vi "Dashboard custom_bartender&global&gripper&camera4.vi"() -> ()   [LabVIEW 2017]
uses:
  C:/Users/IMR Lab/Documents/LabVIEW Data/UniversalRobotsSDK_LABView/LabVIEW/Examples/LabVIEW10/UnderAutomation.UniversalRobots.dll
  UnderAutomation.UniversalRobots.dll
  Global 1.vi
panel:
  in  "stop":bool
  out "3rd Order":bool
  out "2nd Order":bool
  out "1st Order":bool
  out "Rx":dbl
  out "Rz":dbl
  out "Ry":dbl
  out "Enabled":bool
  out "Port":i32
  in  "Move to particular posture":bool
  in  "Move to Zero position":bool
  out "Connected":bool
  in  "Robot IP(192.168.112.182)":string
  out "Connect error":errorcluster
  in  "Power on\nRelease brake":bool
  in  "Power off":bool
  in  "Connect":bool
  in  "Send script":bool
  in  "Script to execute":string
  out "Powered on":bool
  out "X":dbl
  out "Y":dbl
  out "Z":dbl
  out "License state":string
  # "e"
  # "movej( get_inverse_kin(p[0.3138, 0.0814, 0.1647, 0.4226, -2.3876, -2.3851]),  a=0.5, v=0.25, t=0, r=0)"
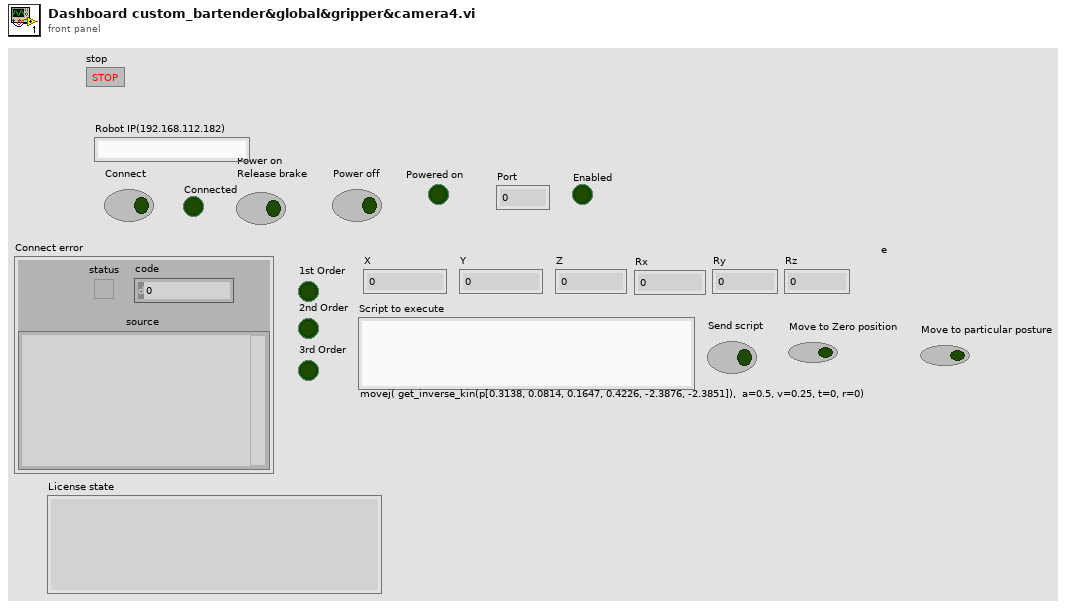
[diagram p1: front panel]
types:
  T1 = enum16{"Standard", "Buffered", "CRLF", "Immediate"}
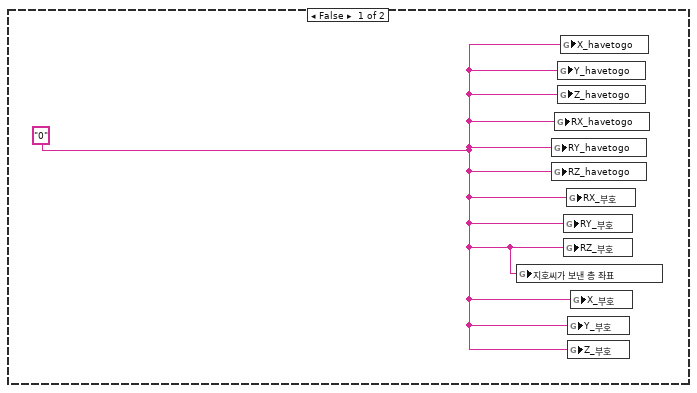
[diagram p2: hidden frame]
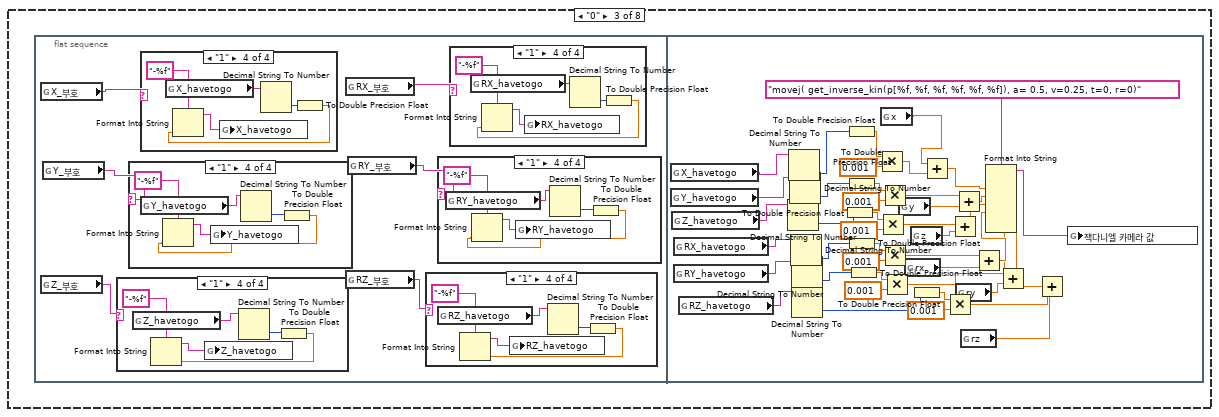
[diagram p5: hidden frame]
diagram:
  w6 = ""
  # "짐빔에서 우유이동 준비 자세"
  # "우유 들어올리는 자세"
  # "우유로 가는 자세"
  # "우유 보는 자세"
  # "술잔 따르는 자세3"
  # "미니콜라 따르는 자세"
  # "술잔 중간지점 가는 자세"
  # "짐빔에서 토닉이동 준비 자세"
  # "술잔 따르는 자세2"
  # "술잔 위로 가는 자세2"
  # "토닉워터 뺴는 자세"
  # "토닉워 들어올리는 자세"
  # "토닉워터 가는 자세"
  # "토닉워터 보는 자세"
  # "짐빔 들어올리는 자세"
  # "짐빔로 가는 자세"
  # "짐빔 보는 자세"
  # "콜라 뺴는 자세"
  # "콜라 들어올리는 자세"
  # "콜라로 가는 자세"
  # "콜라 보는 자세"
  # "술잔 따르는 자세"
  # "술잔 위로 가는 자세"
  # "잭다니엘 들어올리는 자세"
  # "잭다니엘 위치로 가는 자세"
  # "잭다니엘 보는 자세"
  # "1자로 서는 자세"
  # "Example : Display power on status"
  # "Create a UR\ncobot instance"
  # "Show license state"
  # "Register your confidential license key to exit\ntrial period and use this library forever"
  # "Power off when button is clicked"
  # "Power on and release brake when button is clicked"
  # "Get your UR Dashboard interface"
  n1 = global write "Global 1.vi" "술따르는자세2-2"("movej( get_inverse_kin(p[-0.114997, -0.200333, 0.241627, 0.772074, 1.70292, -1.57709]), a= 0.5, v=0.25, t=0, r=0)") -> ()
  n2 = global write "Global 1.vi" "TCP 스위치"(FALSE ("TCP 스위치")) -> ()
  n3 = global write "Global 1.vi" "미니콜라 따르는 자세"("movej([-0.0902,-1.8120,-1.9241,-3.5769,6.2827,8.4658], a=0.5, v=0.25, t=0, r=0)") -> ()
  n4 = global write "Global 1.vi" "짐빔에서 우유준비자세"("movej( get_inverse_kin(p[-0.226891, 0.162413, 0.418489, -0.313613, 2.00693, 1.9348]), a= 0.5, v=0.25, t=0, r=0)") -> ()
  n5 = global write "Global 1.vi" "잭다니엘 들어올리는 자세"("movej([0.8116,-2.0223,-1.2828,-3.0107,4.3284,5.9341], a=0.5, v=0.25, t=0, r=0)") -> ()
  n6 = global write "Global 1.vi" "짐빔 토닉 이동 준비자세"("movej([-0.5421,-0.8131,0.8439,-0.0538,2.5052,5.9032], a=0.5, v=0.25, t=0, r=0)") -> ()
  n7 = global write "Global 1.vi" "우유로 가는 자세"("movej( get_inverse_kin(p[-0.0922578, 0.258702, 0.0945584, -0.185663, 1.9856, 1.89851]), a= 0.5, v=0.25, t=0, r=0)") -> ()
  n8 = global write "Global 1.vi" "우유드는자세"("movej( get_inverse_kin(p[-0.0942522, 0.213042, 0.40064, -0.176149, 1.92162, 1.97243]), a= 0.5, v=0.25, t=0, r=0)") -> ()
  n9 = global write "Global 1.vi" "우유보는자세"("movej( get_inverse_kin(p[-0.103424, 0.183937, 0.100861, -0.211125, 2.02982, 1.84622]), a= 0.5, v=0.25, t=0, r=0)") -> ()
  n10 = global write "Global 1.vi" "토닉 빼는 자세"("movej([-0.5277,-1.5104,1.5889,-0.0548,2.5728,5.9025], a=0.5, v=0.25, t=0, r=0)") -> ()
  n11 = global write "Global 1.vi" "잭다닐 위치로 가는 자세"("movej([0.8116,-2.3119,-1.606,-2.3958,4.3284,5.9341], a=0.5, v=0.25, t=0, r=0)") -> ()
  n12 = global write "Global 1.vi" "토닉 드는 자세"("movej([-1.0311,-1.1460,1.5830,-0.4348,2.0708,5.9048], a=0.5, v=0.25, t=0, r=0)") -> ()
  n13 = global write "Global 1.vi" "토닉 보는 자세"("movej([-0.4690,-1.1292,2.1508,-1.0119,2.6124,5.9032], a=0.5, v=0.25, t=0, r=0)") -> ()
  n14 = global write "Global 1.vi" "술잔 위로 가는 자세 2"("movej([0.0485,-1.6015,2.5780,-1.0382,-0.0520,5.3649], a=0.5, v=0.25, t=0, r=0)") -> ()
  n15 = global write "Global 1.vi" "1자로 서는 자세"("movej([3.1412,-1.5708,0,-1.5708,3.1412,5.8904], a=0.5, v=0.25, t=0, r=0)") -> ()
  n16 = global write "Global 1.vi" "짐빔 들어올리는 자세"("movej([-0.5421,-0.8131,0.8439,-0.0538,2.5052,5.9032], a=0.5, v=0.25, t=0, r=0)") -> ()
  n17 = global write "Global 1.vi" "술잔 위로 가는 자세"("movej([-0.0903,-2.0548,-2.0169,-3.3289,6.2826,7.4091], a=0.5, v=0.25, t=0, r=0)") -> ()
  n18 = global write "Global 1.vi" "토닉 가는자세"("movej([-0.9924,-0.8742,1.7459,-0.8837,2.0958,5.9048], a=0.5, v=0.25, t=0, r=0)") -> ()
  n19 = global write "Global 1.vi" "잭다니엘 보는 자세"("movej([0,-2.2170,-1.4226,-2.2842,3.1412,6.2832], a=0.5, v=0.25, t=0, r=0)") -> ()
  n20 = global write "Global 1.vi" "짐빔 위치로 가는 자세"("movej([-0.5436,-0.4519,0.8428,-0.3534,2.6134,5.9032], a=0.5, v=0.25, t=0, r=0)") -> ()
  n21 = global write "Global 1.vi" "콜라 보는 자세"("movej([0,-1.8110,-2.1684,-2.3033,3.1543,5.9213], a=0.5, v=0.25, t=0, r=0)") -> ()
  n22 = global write "Global 1.vi" "콜라로 가는자세"("movej([1.2020,-2.166,-1.9385,-2.1863,4.3172,5.9210], a=0.5, v=0.25, t=0, r=0)") -> ()
  n23 = global write "Global 1.vi" "콜라 빼는 자세"("movej([0.8789,-1.5237,-2.1070,-2.6679, 3.9917,5.9085], a=0.5, v=0.25, t=0, r=0)") -> ()
  n24 = global write "Global 1.vi" "콜라 드는 자세"("movej([1.2020,-1.8452,-1.7403,-2.7082,4.3162,5.9158], a=0.5, v=0.25, t=0, r=0)") -> ()
  n25 = global write "Global 1.vi" "술 따르는 자세 2"("movej([0.0412,-1.9708,2.4700,-1.0157,-0.0618,4.8998], a=0.5, v=0.25, t=0, r=0)") -> ()
  n26 = global write "Global 1.vi" "잭다니엘 카메라 값"(w6) -> ()
  n27 = global write "Global 1.vi" "술 따르는 자세"("movej([-0.0902,-1.9024,-1.9241,-3.5769,6.2827,8.4692], a=0.5, v=0.25, t=0, r=0)") -> ()
  n28 = global write "Global 1.vi" "짐빔 보는 자세"("movej([-0.0364,-0.6154,0.9421,-0.3291,3.1047,5.9020], a=0.5, v=0.25, t=0, r=0)") -> ()
  n29 = global write "Global 1.vi" "콜라 카메라 값"(w6) -> ()
  n30 = global write "Global 1.vi" "토닉 카메라 값"(w6) -> ()
  n31 = global write "Global 1.vi" "짐빔 카메라 값"(w6) -> ()
  n32 = constructor class="UR"() -> (reference out=w32:refnum<k24>)  [unwired: 3 in, 2 out]
  n33 = global write "Global 1.vi" "술잔 중간지점"("movej([-0.2173,-1.9485,-1.6874,-3.9352,6.2671,7.2276], a=0.5, v=0.25, t=0, r=0)") -> ()
  n34 = while {
    tunnel: w32 -> [w38]
    stop <- FALSE stop-if-true
    # "Connect to the robot when button is pressed"
    # "Show if primary interface is connected"
    # "Get your UR primary interface"
    n35 = property class="UR"(reference=w38) -> ("PrimaryInterface"=w41:refnum<k24>)  [unwired: 1 in, 2 out]
    n36 = Wait (ms)(milliseconds to wait=u32 50) -> ()  [unwired: 1 out]
    n37 = property class="PrimaryInterfaceClientInternal"(reference=w41) -> ("Connected"=w40:bool)  [unwired: 1 in, 2 out]
    "Connected" <- w40
    n38 = case shown="True" "Connect" {
      tunnel: w38 -> [_ w708]
      frame False {
      }
      frame True {
        n39 = flat-sequence {
          tunnel: w708 -> [w710]
          frame #0 {
            n40 = invoke class="UR" method="Connect"(reference=w710, "ip"="Robot IP(192.168.112.182)") -> (error out=→"Connect error":errorcluster)  [unwired: 2 in, 3 out]
          }
        }
      }
    }
    n41 = case shown="True" w40 {
      tunnel: w41 -> [_ w54]
      frame False {
        (unwired) 0.0 ("Rx")
        (unwired) 0.0 ("Rz")
        (unwired) 0.0 ("Ry")
        (unwired) 0.0 ("Z")
        (unwired) 0.0 ("X")
        (unwired) 0.0 ("Y")
      }
      frame True {
        # "Send URScript when button pressed"
        # "Example : Display current cartesian pose"
        n42 = property class="PrimaryInterfaceClientInternal"(reference=w54) -> ("Script"=w55:refnum<k24>)  [unwired: 1 in, 2 out]
        n43 = global read "Global 1.vi" "2nd Order"() -> (w58:bool)
        "2nd Order" <- w58
        n44 = global read "Global 1.vi" "3rd Order"() -> (w57:bool)
        "3rd Order" <- w57
        n45 = global read "Global 1.vi" "1st Order"() -> (w59:bool)
        "1st Order" <- w59
        n46 = Build Array(w59, w58, w57) -> (w60:bool[])
        n47 = Boolean Array To Number(Boolean array=w60) -> (number=w56:u32)
        n48 = case shown="100" w56 {
          tunnel: w55 -> [_ w118 w310 _ w494 _ _ _]
          frame 0, Default {
          }
          frame 1 {
            # "잭다 : 콜라 = 1 : 3"
            # "1st order"
            n49 = flat-sequence {
              tunnel: w118 -> [w122]
              tunnel: [w121] -> w117
              tunnel: w117 -> [w126]
              tunnel: [w124] -> w111
              tunnel: w111 -> [w129]
              tunnel: [w129] -> w110
              tunnel: w110 -> [w132]
              tunnel: [w132] -> w89
              tunnel: w89 -> [w136]
              tunnel: [w136] -> w76
              tunnel: w76 -> [w138]
              tunnel: [w138] -> w75
              tunnel: w75 -> [w142]
              tunnel: [w142] -> w77
              tunnel: w77 -> [w143]
              tunnel: [w143] -> w86
              tunnel: w86 -> [w144]
              tunnel: [w144] -> w88
              tunnel: w88 -> [w146]
              tunnel: [w146] -> w87
              tunnel: w87 -> [w151]
              tunnel: [w148] -> w70
              tunnel: w70 -> [w153]
              tunnel: [w153] -> w69
              tunnel: w69 -> [w157]
              tunnel: [w157] -> w109
              tunnel: w109 -> [w160]
              tunnel: [w160] -> w108
              tunnel: w108 -> [w162]
              tunnel: [w161] -> w97
              tunnel: w97 -> [w166]
              tunnel: [w165] -> w96
              tunnel: w96 -> [w170]
              tunnel: [w169] -> w116
              tunnel: w116 -> [w175]
              tunnel: [w173] -> w115
              tunnel: w115 -> [w178]
              tunnel: [w177] -> w95
              tunnel: w95 -> [w182]
              tunnel: [w181] -> w94
              tunnel: [w185] -> w85
              tunnel: w94 -> [w187]
              tunnel: [w189] -> w107
              tunnel: w85 -> [w190]
              tunnel: w107 -> [w195]
              tunnel: [w195] -> w106
              tunnel: w106 -> [w198]
              tunnel: [w198] -> w105
              tunnel: w105 -> [w200]
              tunnel: [w199] -> w80
              tunnel: w80 -> [w204]
              tunnel: [w204] -> w79
              tunnel: w79 -> [w208]
              tunnel: [w208] -> w74
              tunnel: w74 -> [w210]
              tunnel: [w210] -> w73
              tunnel: w73 -> [w214]
              tunnel: [w214] -> w78
              tunnel: w78 -> [w215]
              tunnel: [w215] -> w83
              tunnel: w83 -> [w216]
              tunnel: [w216] -> w82
              tunnel: w82 -> [w218]
              tunnel: [w218] -> w81
              tunnel: [w219] -> w72
              tunnel: w81 -> [w220]
              tunnel: w72 -> [w224]
              tunnel: [w224] -> w71
              tunnel: w71 -> [w227]
              tunnel: [w227] -> w104
              tunnel: w104 -> [w230]
              tunnel: [w230] -> w84
              tunnel: [w231] -> w103
              tunnel: w84 -> [w232]
              tunnel: w103 -> [w236]
              tunnel: [w235] -> w93
              tunnel: w93 -> [w240]
              tunnel: [w239] -> w92
              tunnel: w92 -> [w244]
              tunnel: [w243] -> w114
              tunnel: w114 -> [w248]
              tunnel: [w247] -> w113
              tunnel: w113 -> [w252]
              tunnel: [w251] -> w91
              tunnel: w91 -> [w256]
              tunnel: [w255] -> w90
              tunnel: w90 -> [w260]
              tunnel: [w259] -> w102
              tunnel: w102 -> [w264]
              tunnel: [w263] -> w112
              tunnel: w112 -> [w268]
              tunnel: [w267] -> w100
              tunnel: [w271] -> w101
              tunnel: w100 -> [w271]
              tunnel: [w274] -> w99
              tunnel: w101 -> [w274]
              tunnel: w99 -> [w278]
              tunnel: [w277] -> w98
              tunnel: w98 -> [w281]
              frame #0 {
                # "초기자세"
                n50 = global read "Global 1.vi" "1자로 서는 자세"() -> (w120:string)
                n51 = invoke class="PrimaryInterfaceScript" method="Send"(reference=w122, "script"=w120) -> (reference out=w121:refnum<k24>)  [unwired: 2 in, 3 out]
                n52 = Wait (ms)(milliseconds to wait=u32 15000) -> ()  [unwired: 1 out]
              }
              frame #1 {
                # "잭다니엘 보기"
                n53 = global read "Global 1.vi" "잭다니엘 보는 자세"() -> (w125:string)
                n54 = invoke class="PrimaryInterfaceScript" method="Send"(reference=w126, "script"=w125) -> (reference out=w124:refnum<k24>)  [unwired: 2 in, 3 out]
                n55 = Wait (ms)(milliseconds to wait=u32 17500) -> ()  [unwired: 1 out]
              }
              frame #2 {
                # "그리퍼 열기"
                n56 = global write "Global 1.vi" "그리퍼 열림"(TRUE ("그리퍼 열림")) -> ()
                n57 = Wait (ms)(milliseconds to wait=u32 300) -> ()  [unwired: 1 out]
              }
              frame #3 {
                n58 = global write "Global 1.vi" "그리퍼 열림"(FALSE ("그리퍼 열림")) -> ()
                n59 = Wait (ms)(milliseconds to wait=u32 300) -> ()  [unwired: 1 out]
              }
              frame #4 {
                # "tcp 키는 스위치 보단\n파이썬한테 \n값 보내달라하는\n요청 보내는 걸로 \n바꾸기"
                n60 = global write "Global 1.vi" "몇번 병을 볼것인가"("0" ("몇번 병을 볼것인가")) -> ()
                n61 = global write "Global 1.vi" "TCP 스위치"(TRUE ("그리퍼 열림")) -> ()
                n62 = Wait Until Next ms Multiple(millisecond multiple=u32 1000 ("milliseconds to wait")) -> ()  [unwired: 1 out]
              }
              frame #5 {
                n63 = Wait (ms)(milliseconds to wait=u32 5000) -> ()  [unwired: 1 out]
              }
              frame #6 {
                n64 = global write "Global 1.vi" "몇번 병을 볼것인가"("0" ("몇번 병을 볼것인가")) -> ()
                n65 = global write "Global 1.vi" "TCP 스위치"(TRUE ("그리퍼 열림")) -> ()
                n66 = Wait Until Next ms Multiple(millisecond multiple=u32 1000 ("milliseconds to wait")) -> ()  [unwired: 1 out]
              }
              frame #7 {
              }
              frame #8 {
              }
              frame #9 {
                n67 = Wait (ms)(milliseconds to wait=u32 1000) -> ()  [unwired: 1 out]
              }
              frame #10 {
                # "잭다니엘 위치로 가기"
                n68 = global write "Global 1.vi" "잭다니엘이동해야함"(TRUE ("잭다니엘이동해야함")) -> ()
                n69 = global read "Global 1.vi" "잭다니엘 카메라 값"() -> (w150:string)
                n70 = invoke class="PrimaryInterfaceScript" method="Send"(reference=w151, "script"=w150) -> (reference out=w148:refnum<k24>)  [unwired: 2 in, 3 out]
                n71 = Wait Until Next ms Multiple(millisecond multiple=u32 7000 ("milliseconds to wait")) -> ()  [unwired: 1 out]
              }
              frame #11 {
                n72 = Wait (ms)(milliseconds to wait=u32 5000) -> ()  [unwired: 1 out]
              }
              frame #12 {
                # "그리퍼 닫기"
                n73 = global write "Global 1.vi" "잭다니엘이동해야함"(FALSE ("잭다니엘이동해야함")) -> ()
                n74 = global write "Global 1.vi" "그리퍼 닫힘"(TRUE ("그리퍼 열림")) -> ()
                n75 = Wait (ms)(milliseconds to wait=u32 300) -> ()  [unwired: 1 out]
              }
              frame #13 {
                n76 = global write "Global 1.vi" "그리퍼 닫힘"(FALSE ("그리퍼 열림")) -> ()
                n77 = Wait (ms)(milliseconds to wait=u32 3000) -> ()  [unwired: 1 out]
              }
              frame #14 {
                # "잭다니엘 들기"
                n78 = global read "Global 1.vi" "잭다니엘 들어올리는 자세"() -> (w164:string)
                n79 = invoke class="PrimaryInterfaceScript" method="Send"(reference=w162, "script"=w164) -> (reference out=w161:refnum<k24>)  [unwired: 2 in, 3 out]
                n80 = Wait (ms)(milliseconds to wait=u32 5000) -> ()  [unwired: 1 out]
              }
              frame #15 {
                # "술잔 중간지점으로 이동"
                n81 = global read "Global 1.vi" "술잔 중간지점"() -> (w167:string)
                n82 = invoke class="PrimaryInterfaceScript" method="Send"(reference=w166, "script"=w167) -> (reference out=w165:refnum<k24>)  [unwired: 2 in, 3 out]
                n83 = Wait (ms)(milliseconds to wait=u32 15000) -> ()  [unwired: 1 out]
              }
              frame #16 {
                # "술잔 쪽으로 이동"
                n84 = global read "Global 1.vi" "술잔 위로 가는 자세"() -> (w171:string)
                n85 = invoke class="PrimaryInterfaceScript" method="Send"(reference=w170, "script"=w171) -> (reference out=w169:refnum<k24>)  [unwired: 2 in, 3 out]
                n86 = Wait (ms)(milliseconds to wait=u32 5000) -> ()  [unwired: 1 out]
              }
              frame #17 {
                # "술따르기"
                n87 = global read "Global 1.vi" "술 따르는 자세"() -> (w174:string)
                n88 = invoke class="PrimaryInterfaceScript" method="Send"(reference=w175, "script"=w174) -> (reference out=w173:refnum<k24>)  [unwired: 2 in, 3 out]
                n89 = Wait (ms)(milliseconds to wait=u32 9000) -> ()  [unwired: 1 out]
              }
              frame #18 {
                # "술따르기 중단"
                n90 = global read "Global 1.vi" "술잔 위로 가는 자세"() -> (w179:string)
                n91 = invoke class="PrimaryInterfaceScript" method="Send"(reference=w178, "script"=w179) -> (reference out=w177:refnum<k24>)  [unwired: 2 in, 3 out]
                n92 = Wait (ms)(milliseconds to wait=u32 4000) -> ()  [unwired: 1 out]
              }
              frame #19 {
                # "술잔 중간지점으로 이동"
                n93 = global read "Global 1.vi" "술잔 중간지점"() -> (w183:string)
                n94 = invoke class="PrimaryInterfaceScript" method="Send"(reference=w182, "script"=w183) -> (reference out=w181:refnum<k24>)  [unwired: 2 in, 3 out]
                n95 = Wait (ms)(milliseconds to wait=u32 7000) -> ()  [unwired: 1 out]
              }
              frame #20 {
                # "잭다니엘 들었던 곳으로"
                n96 = global read "Global 1.vi" "잭다니엘 들어올리는 자세"() -> (w186:string)
                n97 = invoke class="PrimaryInterfaceScript" method="Send"(reference=w187, "script"=w186) -> (reference out=w185:refnum<k24>)  [unwired: 2 in, 3 out]
                n98 = Wait (ms)(milliseconds to wait=u32 10000) -> ()  [unwired: 1 out]
              }
              frame #21 {
                # "잭다니엘 내려놓기"
                n99 = global read "Global 1.vi" "잭다닐 위치로 가는 자세"() -> (w192:string)
                n100 = invoke class="PrimaryInterfaceScript" method="Send"(reference=w190, "script"=w192) -> (reference out=w189:refnum<k24>)  [unwired: 2 in, 3 out]
                n101 = Wait (ms)(milliseconds to wait=u32 5000) -> ()  [unwired: 1 out]
              }
              frame #22 {
                # "그리퍼 열기"
                n102 = global write "Global 1.vi" "그리퍼 열림"(TRUE ("그리퍼 열림")) -> ()
                n103 = Wait (ms)(milliseconds to wait=u32 300) -> ()  [unwired: 1 out]
              }
              frame #23 {
                n104 = global write "Global 1.vi" "그리퍼 열림"(FALSE ("그리퍼 열림")) -> ()
                n105 = Wait (ms)(milliseconds to wait=u32 3000) -> ()  [unwired: 1 out]
              }
              frame #24 {
                # "콜라보러가기"
                n106 = global read "Global 1.vi" "콜라 보는 자세"() -> (w202:string)
                n107 = invoke class="PrimaryInterfaceScript" method="Send"(reference=w200, "script"=w202) -> (reference out=w199:refnum<k24>)  [unwired: 2 in, 3 out]
                n108 = Wait (ms)(milliseconds to wait=u32 10000) -> ()  [unwired: 1 out]
              }
              frame #25 {
                n109 = Wait (ms)(milliseconds to wait=u32 1000) -> ()  [unwired: 1 out]
              }
              frame #26 {
                # "tcp 키는 스위치 보단\n파이썬한테 \n값 보내달라하는\n요청 보내는 걸로 \n바꾸기"
                n110 = global write "Global 1.vi" "몇번 병을 볼것인가"("4" ("몇번 병을 볼것인가")) -> ()
                n111 = global write "Global 1.vi" "TCP 스위치"(TRUE ("그리퍼 열림")) -> ()
                n112 = Wait Until Next ms Multiple(millisecond multiple=u32 1000 ("milliseconds to wait")) -> ()  [unwired: 1 out]
              }
              frame #27 {
                n113 = Wait (ms)(milliseconds to wait=u32 5000) -> ()  [unwired: 1 out]
              }
              frame #28 {
                n114 = global write "Global 1.vi" "몇번 병을 볼것인가"("4" ("몇번 병을 볼것인가")) -> ()
                n115 = global write "Global 1.vi" "TCP 스위치"(TRUE ("그리퍼 열림")) -> ()
                n116 = Wait Until Next ms Multiple(millisecond multiple=u32 1000 ("milliseconds to wait")) -> ()  [unwired: 1 out]
              }
              frame #29 {
              }
              frame #30 {
              }
              frame #31 {
                n117 = Wait (ms)(milliseconds to wait=u32 1000) -> ()  [unwired: 1 out]
              }
              frame #32 {
                # "콜라 들러가기"
                n118 = global read "Global 1.vi" "콜라 카메라 값"() -> (w222:string)
                n119 = invoke class="PrimaryInterfaceScript" method="Send"(reference=w220, "script"=w222) -> (reference out=w219:refnum<k24>)  [unwired: 2 in, 3 out]
                n120 = Wait (ms)(milliseconds to wait=u32 8000) -> ()  [unwired: 1 out]
              }
              frame #33 {
                n121 = Wait (ms)(milliseconds to wait=u32 5000) -> ()  [unwired: 1 out]
              }
              frame #34 {
                n122 = global write "Global 1.vi" "그리퍼 닫힘"(TRUE ("그리퍼 열림")) -> ()
                n123 = Wait (ms)(milliseconds to wait=u32 300) -> ()  [unwired: 1 out]
              }
              frame #35 {
                n124 = global write "Global 1.vi" "그리퍼 닫힘"(FALSE ("그리퍼 열림")) -> ()
                n125 = Wait (ms)(milliseconds to wait=u32 3000) -> ()  [unwired: 1 out]
              }
              frame #36 {
                # "콜라 들어올리기"
                n126 = global read "Global 1.vi" "콜라 드는 자세"() -> (w234:string)
                n127 = invoke class="PrimaryInterfaceScript" method="Send"(reference=w232, "script"=w234) -> (reference out=w231:refnum<k24>)  [unwired: 2 in, 3 out]
                n128 = Wait (ms)(milliseconds to wait=u32 5000) -> ()  [unwired: 1 out]
              }
              frame #37 {
                # "콜라 살짝 빼기"
                n129 = global read "Global 1.vi" "콜라 빼는 자세"() -> (w238:string)
                n130 = invoke class="PrimaryInterfaceScript" method="Send"(reference=w236, "script"=w238) -> (reference out=w235:refnum<k24>)  [unwired: 2 in, 3 out]
                n131 = Wait (ms)(milliseconds to wait=u32 5000) -> ()  [unwired: 1 out]
              }
              frame #38 {
                # "술잔 중간지점으로 이동"
                n132 = global read "Global 1.vi" "술잔 중간지점"() -> (w241:string)
                n133 = invoke class="PrimaryInterfaceScript" method="Send"(reference=w240, "script"=w241) -> (reference out=w239:refnum<k24>)  [unwired: 2 in, 3 out]
                n134 = Wait (ms)(milliseconds to wait=u32 15000) -> ()  [unwired: 1 out]
              }
              frame #39 {
                # "술잔으로 이동"
                n135 = global read "Global 1.vi" "술잔 위로 가는 자세"() -> (w246:string)
                n136 = invoke class="PrimaryInterfaceScript" method="Send"(reference=w244, "script"=w246) -> (reference out=w243:refnum<k24>)  [unwired: 2 in, 3 out]
                n137 = Wait (ms)(milliseconds to wait=u32 5000) -> ()  [unwired: 1 out]
              }
              frame #40 {
                # "미니콜라에 따르기"
                n138 = global read "Global 1.vi" "미니콜라 따르는 자세"() -> (w250:string)
                n139 = invoke class="PrimaryInterfaceScript" method="Send"(reference=w248, "script"=w250) -> (reference out=w247:refnum<k24>)  [unwired: 2 in, 3 out]
                n140 = Wait (ms)(milliseconds to wait=u32 11000) -> ()  [unwired: 1 out]
              }
              frame #41 {
                # "술따르기 중단"
                n141 = global read "Global 1.vi" "술잔 위로 가는 자세"() -> (w254:string)
                n142 = invoke class="PrimaryInterfaceScript" method="Send"(reference=w252, "script"=w254) -> (reference out=w251:refnum<k24>)  [unwired: 2 in, 3 out]
                n143 = Wait (ms)(milliseconds to wait=u32 5000) -> ()  [unwired: 1 out]
              }
              frame #42 {
                # "술잔 중간지점으로 이동"
                n144 = global read "Global 1.vi" "술잔 중간지점"() -> (w257:string)
                n145 = invoke class="PrimaryInterfaceScript" method="Send"(reference=w256, "script"=w257) -> (reference out=w255:refnum<k24>)  [unwired: 2 in, 3 out]
                n146 = Wait (ms)(milliseconds to wait=u32 7000) -> ()  [unwired: 1 out]
              }
              frame #43 {
                # "콜라 뻇던 자세로 복귀"
                n147 = global read "Global 1.vi" "콜라 빼는 자세"() -> (w261:string)
                n148 = invoke class="PrimaryInterfaceScript" method="Send"(reference=w260, "script"=w261) -> (reference out=w259:refnum<k24>)  [unwired: 2 in, 3 out]
                n149 = Wait (ms)(milliseconds to wait=u32 7000) -> ()  [unwired: 1 out]
              }
              frame #44 {
                # "콜라 내려놓으러 가기"
                n150 = global read "Global 1.vi" "콜라 드는 자세"() -> (w266:string)
                n151 = invoke class="PrimaryInterfaceScript" method="Send"(reference=w264, "script"=w266) -> (reference out=w263:refnum<k24>)  [unwired: 2 in, 3 out]
                n152 = Wait (ms)(milliseconds to wait=u32 10000) -> ()  [unwired: 1 out]
              }
              frame #45 {
                # "콜라 내려놓기"
                n153 = global read "Global 1.vi" "콜라로 가는자세"() -> (w270:string)
                n154 = invoke class="PrimaryInterfaceScript" method="Send"(reference=w268, "script"=w270) -> (reference out=w267:refnum<k24>)  [unwired: 2 in, 3 out]
                n155 = Wait (ms)(milliseconds to wait=u32 5000) -> ()  [unwired: 1 out]
              }
              frame #46 {
                # "그리퍼 열기"
                n156 = global write "Global 1.vi" "그리퍼 열림"(TRUE ("그리퍼 열림")) -> ()
                n157 = Wait (ms)(milliseconds to wait=u32 300) -> ()  [unwired: 1 out]
              }
              frame #47 {
                n158 = global write "Global 1.vi" "그리퍼 열림"(FALSE ("그리퍼 열림")) -> ()
                n159 = Wait (ms)(milliseconds to wait=u32 3000) -> ()  [unwired: 1 out]
              }
              frame #48 {
                # "콜라 뻇던 자세로 복귀"
                n160 = global read "Global 1.vi" "콜라 빼는 자세"() -> (w279:string)
                n161 = invoke class="PrimaryInterfaceScript" method="Send"(reference=w278, "script"=w279) -> (reference out=w277:refnum<k24>)  [unwired: 2 in, 3 out]
                n162 = Wait (ms)(milliseconds to wait=u32 5000) -> ()  [unwired: 1 out]
              }
              frame #49 {
                # "초기자세"
                n163 = global read "Global 1.vi" "1자로 서는 자세"() -> (w283:string)
                n164 = invoke class="PrimaryInterfaceScript" method="Send"(reference=w281, "script"=w283) -> ()  [unwired: 2 in, 4 out]
                n165 = Wait (ms)(milliseconds to wait=u32 15000) -> ()  [unwired: 1 out]
              }
              frame #50 {
                n166 = global write "Global 1.vi" "그리퍼 닫힘"(TRUE ("그리퍼 열림")) -> ()
                n167 = Wait (ms)(milliseconds to wait=u32 300) -> ()  [unwired: 1 out]
              }
              frame #51 {
                w286 = ""
                # "그리퍼의 앙다문 일자 입"
                n168 = global write "Global 1.vi" "그리퍼 닫힘"(FALSE ("그리퍼 열림")) -> ()
                n169 = Wait (ms)(milliseconds to wait=u32 3000) -> ()  [unwired: 1 out]
                n170 = global write "Global 1.vi" "잭다니엘 카메라 값"(w286) -> ()
                n171 = global write "Global 1.vi" "콜라 카메라 값"(w286) -> ()
                n172 = global write "Global 1.vi" "토닉 카메라 값"(w286) -> ()
                n173 = global write "Global 1.vi" "짐빔 카메라 값"(w286) -> ()
              }
            }
          }
          frame 2 {
            # "짐빔 : 토닉 = 1: 3"
            # "2nd order"
            n174 = flat-sequence {
              tunnel: w310 -> [w339]
              tunnel: [w338] -> w335
              tunnel: w335 -> [w343]
              tunnel: [w341] -> w334
              tunnel: w334 -> [w346]
              tunnel: [w346] -> w333
              tunnel: w333 -> [w349]
              tunnel: [w349] -> w300
              tunnel: w300 -> [w351]
              tunnel: [w351] -> w299
              tunnel: w299 -> [w355]
              tunnel: [w355] -> w298
              tunnel: w298 -> [w357]
              tunnel: [w357] -> w297
              tunnel: w297 -> [w361]
              tunnel: [w361] -> w296
              tunnel: w296 -> [w362]
              tunnel: [w362] -> w307
              tunnel: w307 -> [w363]
              tunnel: [w363] -> w306
              tunnel: w306 -> [w365]
              tunnel: [w365] -> w305
              tunnel: w305 -> [w369]
              tunnel: [w366] -> w292
              tunnel: w292 -> [w371]
              tunnel: [w371] -> w291
              tunnel: w291 -> [w374]
              tunnel: [w374] -> w332
              tunnel: w332 -> [w377]
              tunnel: [w377] -> w331
              tunnel: w331 -> [w379]
              tunnel: [w378] -> w330
              tunnel: w330 -> [w383]
              tunnel: [w382] -> w329
              tunnel: w329 -> [w388]
              tunnel: [w386] -> w328
              tunnel: w328 -> [w391]
              tunnel: [w390] -> w327
              tunnel: w327 -> [w396]
              tunnel: [w394] -> w326
              tunnel: w326 -> [w399]
              tunnel: [w398] -> w325
              tunnel: w325 -> [w404]
              tunnel: [w404] -> w324
              tunnel: w324 -> [w407]
              tunnel: [w407] -> w309
              tunnel: w309 -> [w409]
              tunnel: [w408] -> w308
              tunnel: [w412] -> w304
              tunnel: w308 -> [w413]
              tunnel: w304 -> [w419]
              tunnel: [w419] -> w295
              tunnel: w295 -> [w421]
              tunnel: [w421] -> w294
              tunnel: w294 -> [w425]
              tunnel: [w425] -> w293
              tunnel: w293 -> [w426]
              tunnel: [w426] -> w303
              tunnel: w303 -> [w427]
              tunnel: [w427] -> w302
              tunnel: w302 -> [w429]
              tunnel: [w429] -> w301
              tunnel: w301 -> [w431]
              tunnel: [w430] -> w290
              tunnel: w290 -> [w435]
              tunnel: [w435] -> w289
              tunnel: w289 -> [w438]
              tunnel: [w438] -> w323
              tunnel: w323 -> [w441]
              tunnel: [w441] -> w322
              tunnel: w322 -> [w443]
              tunnel: [w442] -> w321
              tunnel: w321 -> [w447]
              tunnel: [w446] -> w320
              tunnel: w320 -> [w451]
              tunnel: [w450] -> w319
              tunnel: w319 -> [w455]
              tunnel: [w454] -> w318
              tunnel: w318 -> [w459]
              tunnel: [w458] -> w317
              tunnel: w317 -> [w463]
              tunnel: [w462] -> w316
              tunnel: w316 -> [w467]
              tunnel: [w466] -> w315
              tunnel: w315 -> [w471]
              tunnel: [w470] -> w314
              tunnel: [w474] -> w313
              tunnel: w314 -> [w474]
              tunnel: [w477] -> w312
              tunnel: w313 -> [w477]
              tunnel: w312 -> [w481]
              tunnel: [w480] -> w311
              tunnel: w311 -> [w484]
              frame #0 {
                # "초기자세"
                n175 = global read "Global 1.vi" "1자로 서는 자세"() -> (w337:string)
                n176 = invoke class="PrimaryInterfaceScript" method="Send"(reference=w339, "script"=w337) -> (reference out=w338:refnum<k24>)  [unwired: 2 in, 3 out]
                n177 = Wait (ms)(milliseconds to wait=u32 15000) -> ()  [unwired: 1 out]
              }
              frame #1 {
                # "짐빔 보기"
                n178 = global read "Global 1.vi" "짐빔 보는 자세"() -> (w342:string)
                n179 = invoke class="PrimaryInterfaceScript" method="Send"(reference=w343, "script"=w342) -> (reference out=w341:refnum<k24>)  [unwired: 2 in, 3 out]
                n180 = Wait (ms)(milliseconds to wait=u32 17500) -> ()  [unwired: 1 out]
              }
              frame #2 {
                # "그리퍼 열기"
                n181 = global write "Global 1.vi" "그리퍼 열림"(TRUE ("그리퍼 열림")) -> ()
                n182 = Wait (ms)(milliseconds to wait=u32 300) -> ()  [unwired: 1 out]
              }
              frame #3 {
                n183 = global write "Global 1.vi" "그리퍼 열림"(FALSE ("그리퍼 열림")) -> ()
                n184 = Wait (ms)(milliseconds to wait=u32 300) -> ()  [unwired: 1 out]
              }
              frame #4 {
                n185 = Wait (ms)(milliseconds to wait=u32 2000) -> ()  [unwired: 1 out]
              }
              frame #5 {
                # "tcp 키는 스위치 보단\n파이썬한테 \n값 보내달라하는\n요청 보내는 걸로 \n바꾸기"
                n186 = global write "Global 1.vi" "몇번 병을 볼것인가"("2" ("몇번 병을 볼것인가")) -> ()
                n187 = global write "Global 1.vi" "TCP 스위치"(TRUE ("그리퍼 열림")) -> ()
                n188 = Wait Until Next ms Multiple(millisecond multiple=u32 1000 ("milliseconds to wait")) -> ()  [unwired: 1 out]
              }
              frame #6 {
                n189 = Wait (ms)(milliseconds to wait=u32 5000) -> ()  [unwired: 1 out]
              }
              frame #7 {
                # "똥값방지용"
                n190 = global write "Global 1.vi" "몇번 병을 볼것인가"("2" ("몇번 병을 볼것인가")) -> ()
                n191 = global write "Global 1.vi" "TCP 스위치"(TRUE ("그리퍼 열림")) -> ()
                n192 = Wait Until Next ms Multiple(millisecond multiple=u32 1000 ("milliseconds to wait")) -> ()  [unwired: 1 out]
              }
              frame #8 {
              }
              frame #9 {
              }
              frame #10 {
                n193 = Wait (ms)(milliseconds to wait=u32 1000) -> ()  [unwired: 1 out]
              }
              frame #11 {
                # "짐빔 위치로 가기"
                n194 = global read "Global 1.vi" "짐빔 카메라 값"() -> (w368:string)
                n195 = invoke class="PrimaryInterfaceScript" method="Send"(reference=w369, "script"=w368) -> (reference out=w366:refnum<k24>)  [unwired: 2 in, 3 out]
                n196 = Wait Until Next ms Multiple(millisecond multiple=u32 7000 ("milliseconds to wait")) -> ()  [unwired: 1 out]
              }
              frame #12 {
                n197 = Wait (ms)(milliseconds to wait=u32 5000) -> ()  [unwired: 1 out]
              }
              frame #13 {
                # "그리퍼 닫기"
                n198 = global write "Global 1.vi" "그리퍼 닫힘"(TRUE ("그리퍼 열림")) -> ()
                n199 = Wait (ms)(milliseconds to wait=u32 300) -> ()  [unwired: 1 out]
              }
              frame #14 {
                n200 = global write "Global 1.vi" "그리퍼 닫힘"(FALSE ("그리퍼 열림")) -> ()
                n201 = Wait (ms)(milliseconds to wait=u32 3000) -> ()  [unwired: 1 out]
              }
              frame #15 {
                # "짐빔 들기"
                n202 = global read "Global 1.vi" "짐빔 들어올리는 자세"() -> (w381:string)
                n203 = invoke class="PrimaryInterfaceScript" method="Send"(reference=w379, "script"=w381) -> (reference out=w378:refnum<k24>)  [unwired: 2 in, 3 out]
                n204 = Wait (ms)(milliseconds to wait=u32 5000) -> ()  [unwired: 1 out]
              }
              frame #16 {
                # "술잔 쪽으로 이동"
                n205 = global read "Global 1.vi" "술잔 위로 가는 자세 2"() -> (w384:string)
                n206 = invoke class="PrimaryInterfaceScript" method="Send"(reference=w383, "script"=w384) -> (reference out=w382:refnum<k24>)  [unwired: 2 in, 3 out]
                n207 = Wait (ms)(milliseconds to wait=u32 15000) -> ()  [unwired: 1 out]
              }
              frame #17 {
                # "술따르기"
                n208 = global read "Global 1.vi" "술 따르는 자세 2"() -> (w387:string)
                n209 = invoke class="PrimaryInterfaceScript" method="Send"(reference=w388, "script"=w387) -> (reference out=w386:refnum<k24>)  [unwired: 2 in, 3 out]
                n210 = Wait (ms)(milliseconds to wait=u32 9000) -> ()  [unwired: 1 out]
              }
              frame #18 {
                # "술따르기 중단"
                n211 = global read "Global 1.vi" "술잔 위로 가는 자세 2"() -> (w392:string)
                n212 = invoke class="PrimaryInterfaceScript" method="Send"(reference=w391, "script"=w392) -> (reference out=w390:refnum<k24>)  [unwired: 2 in, 3 out]
                n213 = Wait (ms)(milliseconds to wait=u32 4000) -> ()  [unwired: 1 out]
              }
              frame #19 {
                # "짐빔 들었던 곳으로"
                n214 = global read "Global 1.vi" "짐빔 들어올리는 자세"() -> (w395:string)
                n215 = invoke class="PrimaryInterfaceScript" method="Send"(reference=w396, "script"=w395) -> (reference out=w394:refnum<k24>)  [unwired: 2 in, 3 out]
                n216 = Wait (ms)(milliseconds to wait=u32 10000) -> ()  [unwired: 1 out]
              }
              frame #20 {
                # "짐빔 내려놓기"
                n217 = global read "Global 1.vi" "짐빔 위치로 가는 자세"() -> (w401:string)
                n218 = invoke class="PrimaryInterfaceScript" method="Send"(reference=w399, "script"=w401) -> (reference out=w398:refnum<k24>)  [unwired: 2 in, 3 out]
                n219 = Wait (ms)(milliseconds to wait=u32 5000) -> ()  [unwired: 1 out]
              }
              frame #21 {
                # "그리퍼 열기"
                n220 = global write "Global 1.vi" "그리퍼 열림"(TRUE ("그리퍼 열림")) -> ()
                n221 = Wait (ms)(milliseconds to wait=u32 300) -> ()  [unwired: 1 out]
              }
              frame #22 {
                n222 = global write "Global 1.vi" "그리퍼 열림"(FALSE ("그리퍼 열림")) -> ()
                n223 = Wait (ms)(milliseconds to wait=u32 3000) -> ()  [unwired: 1 out]
              }
              frame #23 {
                # "짐빔에서 토닉으로 이동준비"
                n224 = global read "Global 1.vi" "짐빔 토닉 이동 준비자세"() -> (w411:string)
                n225 = invoke class="PrimaryInterfaceScript" method="Send"(reference=w409, "script"=w411) -> (reference out=w408:refnum<k24>)  [unwired: 2 in, 3 out]
                n226 = Wait (ms)(milliseconds to wait=u32 5000) -> ()  [unwired: 1 out]
              }
              frame #24 {
                # "토닉보러가기"
                n227 = global read "Global 1.vi" "토닉 보는 자세"() -> (w415:string)
                n228 = invoke class="PrimaryInterfaceScript" method="Send"(reference=w413, "script"=w415) -> (reference out=w412:refnum<k24>)  [unwired: 2 in, 3 out]
                n229 = Wait (ms)(milliseconds to wait=u32 11000) -> ()  [unwired: 1 out]
              }
              frame #25 {
                # "tcp 키는 스위치 보단\n파이썬한테 \n값 보내달라하는\n요청 보내는 걸로 \n바꾸기"
                n230 = global write "Global 1.vi" "몇번 병을 볼것인가"("3" ("몇번 병을 볼것인가")) -> ()
                n231 = global write "Global 1.vi" "TCP 스위치"(TRUE ("그리퍼 열림")) -> ()
                n232 = Wait Until Next ms Multiple(millisecond multiple=u32 1000 ("milliseconds to wait")) -> ()  [unwired: 1 out]
              }
              frame #26 {
                n233 = Wait (ms)(milliseconds to wait=u32 5000) -> ()  [unwired: 1 out]
              }
              frame #27 {
                # "똥값 방지용"
                n234 = global write "Global 1.vi" "몇번 병을 볼것인가"("3" ("몇번 병을 볼것인가")) -> ()
                n235 = global write "Global 1.vi" "TCP 스위치"(TRUE ("그리퍼 열림")) -> ()
                n236 = Wait Until Next ms Multiple(millisecond multiple=u32 1000 ("milliseconds to wait")) -> ()  [unwired: 1 out]
              }
              frame #28 {
              }
              frame #29 {
              }
              frame #30 {
                n237 = Wait (ms)(milliseconds to wait=u32 1000) -> ()  [unwired: 1 out]
              }
              frame #31 {
                # "토닉 들러가기"
                n238 = global read "Global 1.vi" "토닉 카메라 값"() -> (w433:string)
                n239 = invoke class="PrimaryInterfaceScript" method="Send"(reference=w431, "script"=w433) -> (reference out=w430:refnum<k24>)  [unwired: 2 in, 3 out]
                n240 = Wait Until Next ms Multiple(millisecond multiple=u32 8000 ("milliseconds to wait")) -> ()  [unwired: 1 out]
              }
              frame #32 {
                n241 = Wait (ms)(milliseconds to wait=u32 5000) -> ()  [unwired: 1 out]
              }
              frame #33 {
                n242 = global write "Global 1.vi" "그리퍼 닫힘"(TRUE ("그리퍼 열림")) -> ()
                n243 = Wait (ms)(milliseconds to wait=u32 300) -> ()  [unwired: 1 out]
              }
              frame #34 {
                n244 = global write "Global 1.vi" "그리퍼 닫힘"(FALSE ("그리퍼 열림")) -> ()
                n245 = Wait (ms)(milliseconds to wait=u32 3000) -> ()  [unwired: 1 out]
              }
              frame #35 {
                # "토닉 들어올리기"
                n246 = global read "Global 1.vi" "토닉 드는 자세"() -> (w445:string)
                n247 = invoke class="PrimaryInterfaceScript" method="Send"(reference=w443, "script"=w445) -> (reference out=w442:refnum<k24>)  [unwired: 2 in, 3 out]
                n248 = Wait (ms)(milliseconds to wait=u32 5000) -> ()  [unwired: 1 out]
              }
              frame #36 {
                # "토닉 살짝 빼기"
                n249 = global read "Global 1.vi" "토닉 빼는 자세"() -> (w449:string)
                n250 = invoke class="PrimaryInterfaceScript" method="Send"(reference=w447, "script"=w449) -> (reference out=w446:refnum<k24>)  [unwired: 2 in, 3 out]
                n251 = Wait (ms)(milliseconds to wait=u32 7000) -> ()  [unwired: 1 out]
              }
              frame #37 {
                # "술잔으로 이동"
                n252 = global read "Global 1.vi" "술잔 위로 가는 자세 2"() -> (w453:string)
                n253 = invoke class="PrimaryInterfaceScript" method="Send"(reference=w451, "script"=w453) -> (reference out=w450:refnum<k24>)  [unwired: 2 in, 3 out]
                n254 = Wait (ms)(milliseconds to wait=u32 12000) -> ()  [unwired: 1 out]
              }
              frame #38 {
                # "술잔에 따르기"
                n255 = global read "Global 1.vi" "술 따르는 자세 2"() -> (w457:string)
                n256 = invoke class="PrimaryInterfaceScript" method="Send"(reference=w455, "script"=w457) -> (reference out=w454:refnum<k24>)  [unwired: 2 in, 3 out]
                n257 = Wait (ms)(milliseconds to wait=u32 13000) -> ()  [unwired: 1 out]
              }
              frame #39 {
                # "술따르기 중단"
                n258 = global read "Global 1.vi" "술잔 위로 가는 자세 2"() -> (w461:string)
                n259 = invoke class="PrimaryInterfaceScript" method="Send"(reference=w459, "script"=w461) -> (reference out=w458:refnum<k24>)  [unwired: 2 in, 3 out]
                n260 = Wait (ms)(milliseconds to wait=u32 5000) -> ()  [unwired: 1 out]
              }
              frame #40 {
                # "토닉 뻇던 자세로 복귀"
                n261 = global read "Global 1.vi" "토닉 빼는 자세"() -> (w464:string)
                n262 = invoke class="PrimaryInterfaceScript" method="Send"(reference=w463, "script"=w464) -> (reference out=w462:refnum<k24>)  [unwired: 2 in, 3 out]
                n263 = Wait (ms)(milliseconds to wait=u32 9000) -> ()  [unwired: 1 out]
              }
              frame #41 {
                # "토닉 내려놓으러 가기"
                n264 = global read "Global 1.vi" "토닉 드는 자세"() -> (w469:string)
                n265 = invoke class="PrimaryInterfaceScript" method="Send"(reference=w467, "script"=w469) -> (reference out=w466:refnum<k24>)  [unwired: 2 in, 3 out]
                n266 = Wait (ms)(milliseconds to wait=u32 7000) -> ()  [unwired: 1 out]
              }
              frame #42 {
                # "토닉 내려놓기"
                n267 = global read "Global 1.vi" "토닉 가는자세"() -> (w473:string)
                n268 = invoke class="PrimaryInterfaceScript" method="Send"(reference=w471, "script"=w473) -> (reference out=w470:refnum<k24>)  [unwired: 2 in, 3 out]
                n269 = Wait (ms)(milliseconds to wait=u32 5000) -> ()  [unwired: 1 out]
              }
              frame #43 {
                # "그리퍼 열기"
                n270 = global write "Global 1.vi" "그리퍼 열림"(TRUE ("그리퍼 열림")) -> ()
                n271 = Wait (ms)(milliseconds to wait=u32 300) -> ()  [unwired: 1 out]
              }
              frame #44 {
                n272 = global write "Global 1.vi" "그리퍼 열림"(FALSE ("그리퍼 열림")) -> ()
                n273 = Wait (ms)(milliseconds to wait=u32 3000) -> ()  [unwired: 1 out]
              }
              frame #45 {
                # "토닉 뻇던 자세로 복귀"
                n274 = global read "Global 1.vi" "토닉 빼는 자세"() -> (w482:string)
                n275 = invoke class="PrimaryInterfaceScript" method="Send"(reference=w481, "script"=w482) -> (reference out=w480:refnum<k24>)  [unwired: 2 in, 3 out]
                n276 = Wait (ms)(milliseconds to wait=u32 5000) -> ()  [unwired: 1 out]
              }
              frame #46 {
                # "초기자세"
                n277 = global read "Global 1.vi" "1자로 서는 자세"() -> (w486:string)
                n278 = invoke class="PrimaryInterfaceScript" method="Send"(reference=w484, "script"=w486) -> ()  [unwired: 2 in, 4 out]
                n279 = Wait (ms)(milliseconds to wait=u32 15000) -> ()  [unwired: 1 out]
              }
              frame #47 {
                n280 = global write "Global 1.vi" "그리퍼 닫힘"(TRUE ("그리퍼 열림")) -> ()
                n281 = Wait (ms)(milliseconds to wait=u32 300) -> ()  [unwired: 1 out]
              }
              frame #48 {
                w489 = ""
                # "그리퍼의 앙다문 일자 입"
                n282 = global write "Global 1.vi" "그리퍼 닫힘"(FALSE ("그리퍼 열림")) -> ()
                n283 = Wait (ms)(milliseconds to wait=u32 3000) -> ()  [unwired: 1 out]
                n284 = global write "Global 1.vi" "잭다니엘 카메라 값"(w489) -> ()
                n285 = global write "Global 1.vi" "콜라 카메라 값"(w489) -> ()
                n286 = global write "Global 1.vi" "토닉 카메라 값"(w489) -> ()
                n287 = global write "Global 1.vi" "짐빔 카메라 값"(w489) -> ()
              }
            }
          }
          frame 3 {
            # "multi order"
          }
          frame 4 {
            # "짐빔 : 우유 = 1 : 3"
            # "3rd order"
            n288 = flat-sequence {
              tunnel: w494 -> [w543]
              tunnel: [w542] -> w539
              tunnel: w539 -> [w547]
              tunnel: [w545] -> w538
              tunnel: w538 -> [w550]
              tunnel: [w550] -> w537
              tunnel: w537 -> [w553]
              tunnel: [w553] -> w536
              tunnel: w536 -> [w555]
              tunnel: [w555] -> w535
              tunnel: w535 -> [w559]
              tunnel: [w559] -> w534
              tunnel: w534 -> [w561]
              tunnel: [w561] -> w533
              tunnel: w533 -> [w565]
              tunnel: [w565] -> w532
              tunnel: w532 -> [w566]
              tunnel: [w566] -> w531
              tunnel: w531 -> [w567]
              tunnel: [w567] -> w530
              tunnel: w530 -> [w569]
              tunnel: [w569] -> w529
              tunnel: w529 -> [w573]
              tunnel: [w570] -> w528
              tunnel: w528 -> [w575]
              tunnel: [w575] -> w527
              tunnel: w527 -> [w578]
              tunnel: [w578] -> w526
              tunnel: w526 -> [w581]
              tunnel: [w581] -> w525
              tunnel: w525 -> [w583]
              tunnel: [w582] -> w524
              tunnel: w524 -> [w587]
              tunnel: [w586] -> w523
              tunnel: w523 -> [w592]
              tunnel: [w590] -> w522
              tunnel: w522 -> [w595]
              tunnel: [w594] -> w521
              tunnel: w521 -> [w600]
              tunnel: [w598] -> w520
              tunnel: w520 -> [w603]
              tunnel: [w602] -> w519
              tunnel: w519 -> [w608]
              tunnel: [w608] -> w518
              tunnel: w518 -> [w611]
              tunnel: [w611] -> w493
              tunnel: w493 -> [w613]
              tunnel: [w612] -> w492
              tunnel: w492 -> [w617]
              tunnel: [w616] -> w517
              tunnel: [w620] -> w516
              tunnel: w517 -> [w621]
              tunnel: w516 -> [w627]
              tunnel: [w627] -> w515
              tunnel: w515 -> [w629]
              tunnel: [w629] -> w514
              tunnel: w514 -> [w633]
              tunnel: [w633] -> w513
              tunnel: w513 -> [w634]
              tunnel: [w634] -> w512
              tunnel: w512 -> [w635]
              tunnel: [w635] -> w511
              tunnel: w511 -> [w637]
              tunnel: [w637] -> w510
              tunnel: w510 -> [w639]
              tunnel: [w638] -> w509
              tunnel: w509 -> [w643]
              tunnel: [w643] -> w508
              tunnel: w508 -> [w646]
              tunnel: [w646] -> w507
              tunnel: w507 -> [w649]
              tunnel: [w649] -> w506
              tunnel: w506 -> [w651]
              tunnel: [w650] -> w505
              tunnel: w505 -> [w654]
              tunnel: [w654] -> w504
              tunnel: w504 -> [w656]
              tunnel: [w655] -> w503
              tunnel: w503 -> [w660]
              tunnel: [w659] -> w502
              tunnel: w502 -> [w664]
              tunnel: [w663] -> w501
              tunnel: w501 -> [w667]
              tunnel: [w667] -> w500
              tunnel: w500 -> [w669]
              tunnel: [w668] -> w499
              tunnel: w499 -> [w673]
              tunnel: [w672] -> w498
              tunnel: [w676] -> w497
              tunnel: w498 -> [w676]
              tunnel: [w679] -> w496
              tunnel: w497 -> [w679]
              tunnel: w496 -> [w683]
              tunnel: [w682] -> w495
              tunnel: w495 -> [w686]
              frame #0 {
                # "초기자세"
                n289 = global read "Global 1.vi" "1자로 서는 자세"() -> (w541:string)
                n290 = invoke class="PrimaryInterfaceScript" method="Send"(reference=w543, "script"=w541) -> (reference out=w542:refnum<k24>)  [unwired: 2 in, 3 out]
                n291 = Wait (ms)(milliseconds to wait=u32 15000) -> ()  [unwired: 1 out]
              }
              frame #1 {
                # "짐빔 보기"
                n292 = global read "Global 1.vi" "짐빔 보는 자세"() -> (w546:string)
                n293 = invoke class="PrimaryInterfaceScript" method="Send"(reference=w547, "script"=w546) -> (reference out=w545:refnum<k24>)  [unwired: 2 in, 3 out]
                n294 = Wait (ms)(milliseconds to wait=u32 17500) -> ()  [unwired: 1 out]
              }
              frame #2 {
                # "그리퍼 열기"
                n295 = global write "Global 1.vi" "그리퍼 열림"(TRUE ("그리퍼 열림")) -> ()
                n296 = Wait (ms)(milliseconds to wait=u32 300) -> ()  [unwired: 1 out]
              }
              frame #3 {
                n297 = global write "Global 1.vi" "그리퍼 열림"(FALSE ("그리퍼 열림")) -> ()
                n298 = Wait (ms)(milliseconds to wait=u32 300) -> ()  [unwired: 1 out]
              }
              frame #4 {
                n299 = Wait (ms)(milliseconds to wait=u32 2000) -> ()  [unwired: 1 out]
              }
              frame #5 {
                # "tcp 키는 스위치 보단\n파이썬한테 \n값 보내달라하는\n요청 보내는 걸로 \n바꾸기"
                n300 = global write "Global 1.vi" "몇번 병을 볼것인가"("2" ("몇번 병을 볼것인가")) -> ()
                n301 = global write "Global 1.vi" "TCP 스위치"(TRUE ("그리퍼 열림")) -> ()
                n302 = Wait Until Next ms Multiple(millisecond multiple=u32 1000 ("milliseconds to wait")) -> ()  [unwired: 1 out]
              }
              frame #6 {
                n303 = Wait (ms)(milliseconds to wait=u32 5000) -> ()  [unwired: 1 out]
              }
              frame #7 {
                # "똥값방지용"
                n304 = global write "Global 1.vi" "몇번 병을 볼것인가"("2" ("몇번 병을 볼것인가")) -> ()
                n305 = global write "Global 1.vi" "TCP 스위치"(TRUE ("그리퍼 열림")) -> ()
                n306 = Wait Until Next ms Multiple(millisecond multiple=u32 1000 ("milliseconds to wait")) -> ()  [unwired: 1 out]
              }
              frame #8 {
              }
              frame #9 {
              }
              frame #10 {
                n307 = Wait (ms)(milliseconds to wait=u32 1000) -> ()  [unwired: 1 out]
              }
              frame #11 {
                # "짐빔 위치로 가기"
                n308 = global read "Global 1.vi" "짐빔 카메라 값"() -> (w572:string)
                n309 = invoke class="PrimaryInterfaceScript" method="Send"(reference=w573, "script"=w572) -> (reference out=w570:refnum<k24>)  [unwired: 2 in, 3 out]
                n310 = Wait Until Next ms Multiple(millisecond multiple=u32 7000 ("milliseconds to wait")) -> ()  [unwired: 1 out]
              }
              frame #12 {
                n311 = Wait (ms)(milliseconds to wait=u32 5000) -> ()  [unwired: 1 out]
              }
              frame #13 {
                # "그리퍼 닫기"
                n312 = global write "Global 1.vi" "그리퍼 닫힘"(TRUE ("그리퍼 열림")) -> ()
                n313 = Wait (ms)(milliseconds to wait=u32 300) -> ()  [unwired: 1 out]
              }
              frame #14 {
                n314 = global write "Global 1.vi" "그리퍼 닫힘"(FALSE ("그리퍼 열림")) -> ()
                n315 = Wait (ms)(milliseconds to wait=u32 3000) -> ()  [unwired: 1 out]
              }
              frame #15 {
                # "짐빔 들기"
                n316 = global read "Global 1.vi" "짐빔 들어올리는 자세"() -> (w585:string)
                n317 = invoke class="PrimaryInterfaceScript" method="Send"(reference=w583, "script"=w585) -> (reference out=w582:refnum<k24>)  [unwired: 2 in, 3 out]
                n318 = Wait (ms)(milliseconds to wait=u32 5000) -> ()  [unwired: 1 out]
              }
              frame #16 {
                # "술잔 쪽으로 이동"
                n319 = global read "Global 1.vi" "술잔 위로 가는 자세 2"() -> (w588:string)
                n320 = invoke class="PrimaryInterfaceScript" method="Send"(reference=w587, "script"=w588) -> (reference out=w586:refnum<k24>)  [unwired: 2 in, 3 out]
                n321 = Wait (ms)(milliseconds to wait=u32 15000) -> ()  [unwired: 1 out]
              }
              frame #17 {
                # "술따르기"
                n322 = global read "Global 1.vi" "술따르는자세2-2"() -> (w591:string)
                n323 = invoke class="PrimaryInterfaceScript" method="Send"(reference=w592, "script"=w591) -> (reference out=w590:refnum<k24>)  [unwired: 2 in, 3 out]
                n324 = Wait (ms)(milliseconds to wait=u32 5500) -> ()  [unwired: 1 out]
              }
              frame #18 {
                # "술따르기 중단"
                n325 = global read "Global 1.vi" "술잔 위로 가는 자세 2"() -> (w596:string)
                n326 = invoke class="PrimaryInterfaceScript" method="Send"(reference=w595, "script"=w596) -> (reference out=w594:refnum<k24>)  [unwired: 2 in, 3 out]
                n327 = Wait (ms)(milliseconds to wait=u32 4000) -> ()  [unwired: 1 out]
              }
              frame #19 {
                # "짐빔 들었던 곳으로"
                n328 = global read "Global 1.vi" "짐빔 들어올리는 자세"() -> (w599:string)
                n329 = invoke class="PrimaryInterfaceScript" method="Send"(reference=w600, "script"=w599) -> (reference out=w598:refnum<k24>)  [unwired: 2 in, 3 out]
                n330 = Wait (ms)(milliseconds to wait=u32 10000) -> ()  [unwired: 1 out]
              }
              frame #20 {
                # "짐빔 내려놓기"
                n331 = global read "Global 1.vi" "짐빔 위치로 가는 자세"() -> (w605:string)
                n332 = invoke class="PrimaryInterfaceScript" method="Send"(reference=w603, "script"=w605) -> (reference out=w602:refnum<k24>)  [unwired: 2 in, 3 out]
                n333 = Wait (ms)(milliseconds to wait=u32 5000) -> ()  [unwired: 1 out]
              }
              frame #21 {
                # "그리퍼 열기"
                n334 = global write "Global 1.vi" "그리퍼 열림"(TRUE ("그리퍼 열림")) -> ()
                n335 = Wait (ms)(milliseconds to wait=u32 300) -> ()  [unwired: 1 out]
              }
              frame #22 {
                n336 = global write "Global 1.vi" "그리퍼 열림"(FALSE ("그리퍼 열림")) -> ()
                n337 = Wait (ms)(milliseconds to wait=u32 3000) -> ()  [unwired: 1 out]
              }
              frame #23 {
                n338 = global read "Global 1.vi" "짐빔 보는 자세"() -> (w614:string)
                n339 = invoke class="PrimaryInterfaceScript" method="Send"(reference=w613, "script"=w614) -> (reference out=w612:refnum<k24>)  [unwired: 2 in, 3 out]
                n340 = Wait (ms)(milliseconds to wait=u32 7000) -> ()  [unwired: 1 out]
              }
              frame #24 {
                # "짐빔에서 우유으로 이동준비"
                n341 = global read "Global 1.vi" "짐빔에서 우유준비자세"() -> (w619:string)
                n342 = invoke class="PrimaryInterfaceScript" method="Send"(reference=w617, "script"=w619) -> (reference out=w616:refnum<k24>)  [unwired: 2 in, 3 out]
                n343 = Wait (ms)(milliseconds to wait=u32 7000) -> ()  [unwired: 1 out]
              }
              frame #25 {
                # "우유보러가기"
                n344 = global read "Global 1.vi" "우유보는자세"() -> (w623:string)
                n345 = invoke class="PrimaryInterfaceScript" method="Send"(reference=w621, "script"=w623) -> (reference out=w620:refnum<k24>)  [unwired: 2 in, 3 out]
                n346 = Wait (ms)(milliseconds to wait=u32 11000) -> ()  [unwired: 1 out]
              }
              frame #26 {
                # "tcp 키는 스위치 보단\n파이썬한테 \n값 보내달라하는\n요청 보내는 걸로 \n바꾸기"
                n347 = global write "Global 1.vi" "몇번 병을 볼것인가"("1" ("몇번 병을 볼것인가")) -> ()
                n348 = global write "Global 1.vi" "TCP 스위치"(TRUE ("그리퍼 열림")) -> ()
                n349 = Wait Until Next ms Multiple(millisecond multiple=u32 1000 ("milliseconds to wait")) -> ()  [unwired: 1 out]
              }
              frame #27 {
                n350 = Wait (ms)(milliseconds to wait=u32 5000) -> ()  [unwired: 1 out]
              }
              frame #28 {
                # "똥값 방지용"
                n351 = global write "Global 1.vi" "몇번 병을 볼것인가"("1" ("몇번 병을 볼것인가")) -> ()
                n352 = global write "Global 1.vi" "TCP 스위치"(TRUE ("그리퍼 열림")) -> ()
                n353 = Wait Until Next ms Multiple(millisecond multiple=u32 1000 ("milliseconds to wait")) -> ()  [unwired: 1 out]
              }
              frame #29 {
              }
              frame #30 {
              }
              frame #31 {
                n354 = Wait (ms)(milliseconds to wait=u32 1000) -> ()  [unwired: 1 out]
              }
              frame #32 {
                # "토닉 들러가기"
                n355 = global read "Global 1.vi" "우유 카메라 값"() -> (w641:string)
                n356 = invoke class="PrimaryInterfaceScript" method="Send"(reference=w639, "script"=w641) -> (reference out=w638:refnum<k24>)  [unwired: 2 in, 3 out]
                n357 = Wait Until Next ms Multiple(millisecond multiple=u32 8000 ("milliseconds to wait")) -> ()  [unwired: 1 out]
              }
              frame #33 {
                n358 = Wait (ms)(milliseconds to wait=u32 5000) -> ()  [unwired: 1 out]
              }
              frame #34 {
                n359 = global write "Global 1.vi" "그리퍼 닫힘"(TRUE ("그리퍼 열림")) -> ()
                n360 = Wait (ms)(milliseconds to wait=u32 300) -> ()  [unwired: 1 out]
              }
              frame #35 {
                n361 = global write "Global 1.vi" "그리퍼 닫힘"(FALSE ("그리퍼 열림")) -> ()
                n362 = Wait (ms)(milliseconds to wait=u32 3000) -> ()  [unwired: 1 out]
              }
              frame #36 {
                # "우유 들어올리기"
                n363 = global read "Global 1.vi" "우유드는자세"() -> (w653:string)
                n364 = invoke class="PrimaryInterfaceScript" method="Send"(reference=w651, "script"=w653) -> (reference out=w650:refnum<k24>)  [unwired: 2 in, 3 out]
                n365 = Wait (ms)(milliseconds to wait=u32 5000) -> ()  [unwired: 1 out]
              }
              frame #37 {
                # "토닉 살짝 빼기"
              }
              frame #38 {
                # "술잔으로 이동"
                n366 = global read "Global 1.vi" "술잔 위로 가는 자세 2"() -> (w658:string)
                n367 = invoke class="PrimaryInterfaceScript" method="Send"(reference=w656, "script"=w658) -> (reference out=w655:refnum<k24>)  [unwired: 2 in, 3 out]
                n368 = Wait (ms)(milliseconds to wait=u32 12000) -> ()  [unwired: 1 out]
              }
              frame #39 {
                # "술잔에 따르기"
                n369 = global read "Global 1.vi" "술 따르는 자세 2"() -> (w662:string)
                n370 = invoke class="PrimaryInterfaceScript" method="Send"(reference=w660, "script"=w662) -> (reference out=w659:refnum<k24>)  [unwired: 2 in, 3 out]
                n371 = Wait (ms)(milliseconds to wait=u32 13000) -> ()  [unwired: 1 out]
              }
              frame #40 {
                # "술따르기 중단"
                n372 = global read "Global 1.vi" "술잔 위로 가는 자세 2"() -> (w666:string)
                n373 = invoke class="PrimaryInterfaceScript" method="Send"(reference=w664, "script"=w666) -> (reference out=w663:refnum<k24>)  [unwired: 2 in, 3 out]
                n374 = Wait (ms)(milliseconds to wait=u32 5000) -> ()  [unwired: 1 out]
              }
              frame #41 {
                # "토닉 뻇던 자세로 복귀"
              }
              frame #42 {
                # "토닉 내려놓으러 가기"
                n375 = global read "Global 1.vi" "우유드는자세"() -> (w671:string)
                n376 = invoke class="PrimaryInterfaceScript" method="Send"(reference=w669, "script"=w671) -> (reference out=w668:refnum<k24>)  [unwired: 2 in, 3 out]
                n377 = Wait (ms)(milliseconds to wait=u32 7000) -> ()  [unwired: 1 out]
              }
              frame #43 {
                # "토닉 내려놓기"
                n378 = global read "Global 1.vi" "우유로 가는 자세"() -> (w675:string)
                n379 = invoke class="PrimaryInterfaceScript" method="Send"(reference=w673, "script"=w675) -> (reference out=w672:refnum<k24>)  [unwired: 2 in, 3 out]
                n380 = Wait (ms)(milliseconds to wait=u32 5000) -> ()  [unwired: 1 out]
              }
              frame #44 {
                # "그리퍼 열기"
                n381 = global write "Global 1.vi" "그리퍼 열림"(TRUE ("그리퍼 열림")) -> ()
                n382 = Wait (ms)(milliseconds to wait=u32 300) -> ()  [unwired: 1 out]
              }
              frame #45 {
                n383 = global write "Global 1.vi" "그리퍼 열림"(FALSE ("그리퍼 열림")) -> ()
                n384 = Wait (ms)(milliseconds to wait=u32 3000) -> ()  [unwired: 1 out]
              }
              frame #46 {
                # "토닉 뻇던 자세로 복귀"
                n385 = global read "Global 1.vi" "우유드는자세"() -> (w684:string)
                n386 = invoke class="PrimaryInterfaceScript" method="Send"(reference=w683, "script"=w684) -> (reference out=w682:refnum<k24>)  [unwired: 2 in, 3 out]
                n387 = Wait (ms)(milliseconds to wait=u32 5000) -> ()  [unwired: 1 out]
              }
              frame #47 {
                # "초기자세"
                n388 = global read "Global 1.vi" "1자로 서는 자세"() -> (w688:string)
                n389 = invoke class="PrimaryInterfaceScript" method="Send"(reference=w686, "script"=w688) -> ()  [unwired: 2 in, 4 out]
                n390 = Wait (ms)(milliseconds to wait=u32 15000) -> ()  [unwired: 1 out]
              }
              frame #48 {
                n391 = global write "Global 1.vi" "그리퍼 닫힘"(TRUE ("그리퍼 열림")) -> ()
                n392 = Wait (ms)(milliseconds to wait=u32 300) -> ()  [unwired: 1 out]
              }
              frame #49 {
                w691 = ""
                # "그리퍼의 앙다문 일자 입"
                n393 = global write "Global 1.vi" "그리퍼 닫힘"(FALSE ("그리퍼 열림")) -> ()
                n394 = Wait (ms)(milliseconds to wait=u32 3000) -> ()  [unwired: 1 out]
                n395 = global write "Global 1.vi" "잭다니엘 카메라 값"(w691) -> ()
                n396 = global write "Global 1.vi" "콜라 카메라 값"(w691) -> ()
                n397 = global write "Global 1.vi" "우유 카메라 값"(w691) -> ()
                n398 = global write "Global 1.vi" "토닉 카메라 값"(w691) -> ()
                n399 = global write "Global 1.vi" "짐빔 카메라 값"(w691) -> ()
              }
            }
          }
          frame 5 {
            # "multi order"
          }
          frame 6 {
            # "multi order"
          }
          frame 7 {
            # "multi order"
          }
        }
        n400 = case shown="True" "Send script" {
          tunnel: w55 -> [_ w700]
          frame False {
          }
          frame True {
            n401 = flat-sequence {
              tunnel: w700 -> [w702]
              frame #0 {
                n402 = invoke class="PrimaryInterfaceScript" method="Send"(reference=w702, "script"="Script to execute") -> ()  [unwired: 2 in, 4 out]
              }
            }
          }
        }
        n403 = case shown="True" "Move to Zero position" {
          tunnel: w55 -> [_ w697]
          frame False {
          }
          frame True {
            n404 = flat-sequence {
              tunnel: w697 -> [w699]
              frame #0 {
                n405 = invoke class="PrimaryInterfaceScript" method="Send"(reference=w699, "script"="movej([3.1412,-1.5708,0,-1.5708,3.1412,5.8904], a=0.5, v=0.25, t=0, r=0)") -> ()  [unwired: 2 in, 4 out]
              }
            }
          }
        }
        n406 = case shown="True" "Move to particular posture" {
          tunnel: w55 -> [_ w694]
          frame False {
          }
          frame True {
            n407 = flat-sequence {
              tunnel: w694 -> [w696]
              frame #0 {
                n408 = invoke class="PrimaryInterfaceScript" method="Send"(reference=w696, "script"="movej([-1.5,-1.5,-2,-0.5,1.8,0], a=1.4, v=1.05, t=0, r=0)") -> ()  [unwired: 2 in, 4 out]
              }
            }
          }
        }
        n409 = property class="PrimaryInterfaceClientInternal"(reference=w54) -> ("RobotModeData"=w67:refnum<k24>)  [unwired: 1 in, 2 out]
        n410 = property class="PrimaryInterfaceClientInternal"(reference=w54) -> ("CartesianInfo"=w53:refnum<k24>)  [unwired: 1 in, 2 out]
        n411 = property class="RobotModeDataPackageEventArgs"(reference=w67) -> ("RobotPowerOn"=→"Powered on":bool)  [unwired: 1 in, 2 out]
        n412 = constructor class="SocketCommunicationServer"() -> (reference out=w63:refnum<k24>)  [unwired: 3 in, 2 out]
        n413 = property class="SocketCommunicationServer"(reference=w63) -> ("Enabled"=→"Enabled":bool)  [unwired: 1 in, 2 out]
        n414 = property class="SocketCommunicationServer"(reference=w63) -> ("Port"=→"Port":i32)  [unwired: 1 in, 2 out]
        n415 = property class="CartesianInfoPackageEventArgs"(reference=w53) -> ("Y"=→"Y":dbl)  [unwired: 1 in, 2 out]
        n416 = property class="CartesianInfoPackageEventArgs"(reference=w53) -> ("Ry"=→"Ry":dbl)  [unwired: 1 in, 2 out]
        n417 = property class="CartesianInfoPackageEventArgs"(reference=w53) -> ("Z"=→"Z":dbl)  [unwired: 1 in, 2 out]
        n418 = property class="CartesianInfoPackageEventArgs"(reference=w53) -> ("Rz"=→"Rz":dbl)  [unwired: 1 in, 2 out]
        n419 = property class="CartesianInfoPackageEventArgs"(reference=w53) -> ("X"=→"X":dbl)  [unwired: 1 in, 2 out]
        n420 = property class="CartesianInfoPackageEventArgs"(reference=w53) -> ("Rx"=→"Rx":dbl)  [unwired: 1 in, 2 out]
      }
    }
    n421 = property class="UR"(reference=w38) -> ("Dashboard"=w42:refnum<k24>)  [unwired: 1 in, 2 out]
    n422 = case shown="True" "Power off" {
      tunnel: w42 -> [_ w703]
      frame False {
      }
      frame True {
        n423 = flat-sequence {
          tunnel: w703 -> [w704]
          frame #0 {
            n424 = invoke class="DashboardClientInternal" method="PowerOff"(reference=w704) -> ()  [unwired: 2 in, 3 out]
          }
        }
      }
    }
    n425 = case shown="True" "Power on\nRelease brake" {
      tunnel: w42 -> [_ w705]
      frame False {
      }
      frame True {
        n426 = flat-sequence {
          tunnel: w705 -> [w707]
          frame #0 {
            n427 = invoke class="DashboardClientInternal" method="PowerOn"(reference=w707) -> (reference out=w706:refnum<k24>)  [unwired: 2 in, 2 out]
            n428 = invoke class="DashboardClientInternal" method="ReleaseBrake"(reference=w706) -> ()  [unwired: 2 in, 3 out]
          }
        }
      }
    }
  }
  n429 = invoke class="UR" method="RegisterLicense"(reference=w32, "licensee"="your company name", "key"="") -> (reference out=w34:refnum<k24>)  [unwired: 2 in, 4 out]
  n430 = control-ref of="Script to execute"() -> (w31:refnum<vi>)
  n431 = property class="Str"(reference=w31, "Value"="movej([-1.5,-1.5,-2,-0.5,1.8,0], a=1.4, v=1.05, t=0, r=0)") -> ()  [unwired: 1 in, 2 out]
  n432 = property class="UR"(reference=w34) -> ("LicenseInfo"=w33:refnum<k24>)  [unwired: 1 in, 2 out]
  n433 = invoke class="LicenseInfo" method="ToString"(reference=w33) -> ("ToString"=→"License state":string)  [unwired: 2 in, 2 out]
  n434 = while {
    stop <- "stop" stop-if-true
    n435 = global read "Global 1.vi" "TCP 스위치"() -> (w714:bool)
    n436 = case shown="True" w714 {
      frame False {
        w715 = "0"
        n437 = global write "Global 1.vi" "지호씨가 보낸 총 좌표"(w715) -> ()
        n438 = global write "Global 1.vi" "RY_havetogo"(w715) -> ()
        n439 = global write "Global 1.vi" "RZ_havetogo"(w715) -> ()
        n440 = global write "Global 1.vi" "RX_havetogo"(w715) -> ()
        n441 = global write "Global 1.vi" "Y_havetogo"(w715) -> ()
        n442 = global write "Global 1.vi" "Z_havetogo"(w715) -> ()
        n443 = global write "Global 1.vi" "X_havetogo"(w715) -> ()
        n444 = global write "Global 1.vi" "RY_부호"(w715) -> ()
        n445 = global write "Global 1.vi" "RZ_부호"(w715) -> ()
        n446 = global write "Global 1.vi" "RX_부호"(w715) -> ()
        n447 = global write "Global 1.vi" "Y_부호"(w715) -> ()
        n448 = global write "Global 1.vi" "Z_부호"(w715) -> ()
        n449 = global write "Global 1.vi" "X_부호"(w715) -> ()
      }
      frame True {
        n450 = flat-sequence {
          frame #0 {
            w752 = 4 ("length (rest)")
            n451 = global read "Global 1.vi" "몇번 병을 볼것인가"() -> (w743:string)
            n452 = TCP Open Connection(address="192.168.112.18", remote port or service name=u16 8089) -> (connection ID=w747:refnum<k5>, error out=w746:errorcluster)  [unwired: 3 in]
            n453 = TCP Write(connection ID=w747, data in=w743, error in (no error)=w746) -> (connection ID out=w745:refnum<k5>, error out=w744:errorcluster)  [unwired: 1 in, 1 out]
            n454 = TCP Read(connection ID=w745, bytes to read=30, error in (no error)=w744, 7:T1."Buffered" ("mode (standard)")) -> (connection ID out=w756:refnum<k5>, data out=w716:string, error out=w755:errorcluster)  [unwired: 1 in]
            n455 = String Subset(string=w716, offset (0)=11, length (rest)=w752) -> (substring=w734:string)
            n456 = String Subset(string=w716, offset (0)=16, length (rest)=w752) -> (substring=w733:string)
            n457 = String Subset(string=w716, offset (0)=6, length (rest)=w752) -> (substring=w735:string)
            n458 = String Subset(string=w716, offset (0)=1, length (rest)=w752) -> (substring=w736:string)
            n459 = global write "Global 1.vi" "X_havetogo"(w736) -> ()
            n460 = global write "Global 1.vi" "Z_havetogo"(w734) -> ()
            n461 = global write "Global 1.vi" "RX_havetogo"(w733) -> ()
            n462 = global write "Global 1.vi" "Y_havetogo"(w735) -> ()
            n463 = String Subset(string=w716, offset (0)=26, length (rest)=w752) -> (substring=w731:string)
            n464 = String Subset(string=w716, offset (0)=21, length (rest)=w752) -> (substring=w732:string)
            n465 = global write "Global 1.vi" "지호씨가 보낸 총 좌표"(w716) -> ()
            n466 = String Subset(string=w716, offset (0)=20, length (rest)=1 ("length (rest)")) -> (substring=w729:string)
            n467 = String Subset(string=w716, offset (0)=15, length (rest)=1 ("length (rest)")) -> (substring=w730:string)
            n468 = String Subset(string=w716, offset (0)=25, length (rest)=1 ("length (rest)")) -> (substring=w728:string)
            n469 = global write "Global 1.vi" "RY_havetogo"(w732) -> ()
            n470 = TCP Close Connection(connection ID=w756, error in (no error)=w755) -> ()  [unwired: 1 in, 2 out]
            n471 = global write "Global 1.vi" "RZ_havetogo"(w731) -> ()
            n472 = global write "Global 1.vi" "RY_부호"(w729) -> ()
            n473 = global write "Global 1.vi" "RX_부호"(w730) -> ()
            n474 = global write "Global 1.vi" "RZ_부호"(w728) -> ()
            n475 = String Subset(string=w716, offset (0)=0, length (rest)=1 ("length (rest)")) -> (substring=w725:string)
            n476 = String Subset(string=w716, offset (0)=5, length (rest)=1 ("length (rest)")) -> (substring=w722:string)
            n477 = String Subset(string=w716, offset (0)=10, length (rest)=1 ("length (rest)")) -> (substring=w719:string)
            n478 = global write "Global 1.vi" "X_부호"(w725) -> ()
            n479 = global write "Global 1.vi" "Y_부호"(w722) -> ()
            n480 = global write "Global 1.vi" "Z_부호"(w719) -> ()
          }
          frame #1 {
            n481 = global read "Global 1.vi" "몇번 병을 볼것인가"() -> (w759:string)
            n482 = case shown="\"1\"" w759 {
              frame "False", Default {
              }
              frame "True" {
              }
              frame "0" {
                n483 = flat-sequence {
                  frame #0 {
                    n484 = global read "Global 1.vi" "X_부호"() -> (w762:string)
                    n485 = global read "Global 1.vi" "Z_부호"() -> (w760:string)
                    n486 = global read "Global 1.vi" "Y_부호"() -> (w761:string)
                    n487 = case shown="\"1\"" w760 {
                      frame "False", Default {
                      }
                      frame "True" {
                      }
                      frame "2" {
                      }
                      frame "1" {
                        n488 = global read "Global 1.vi" "Z_havetogo"() -> (w767:string)
                        n489 = Decimal String To Number(string=w767) -> (number=w770:i32)  [unwired: 2 in, 1 out]
                        n490 = To Double Precision Float(number=w770) -> (double precision float=w769:dbl)
                        n491 = Format Into String(format string="-%f", w769) -> (resulting string=w766:string)  [unwired: 2 in, 1 out]
                        n492 = global write "Global 1.vi" "Z_havetogo"(w766) -> ()
                      }
                    }
                    n493 = case shown="\"1\"" w761 {
                      frame "False", Default {
                      }
                      frame "True" {
                      }
                      frame "2" {
                      }
                      frame "1" {
                        n494 = global read "Global 1.vi" "Y_havetogo"() -> (w772:string)
                        n495 = Decimal String To Number(string=w772) -> (number=w775:i32)  [unwired: 2 in, 1 out]
                        n496 = To Double Precision Float(number=w775) -> (double precision float=w773:dbl)
                        n497 = Format Into String(format string="-%f", w773) -> (resulting string=w771:string)  [unwired: 2 in, 1 out]
                        n498 = global write "Global 1.vi" "Y_havetogo"(w771) -> ()
                      }
                    }
                    n499 = case shown="\"1\"" w762 {
                      frame "False", Default {
                      }
                      frame "True" {
                      }
                      frame "2" {
                      }
                      frame "1" {
                        n500 = global read "Global 1.vi" "X_havetogo"() -> (w777:string)
                        n501 = Decimal String To Number(string=w777) -> (number=w780:i32)  [unwired: 2 in, 1 out]
                        n502 = To Double Precision Float(number=w780) -> (double precision float=w779:dbl)
                        n503 = Format Into String(format string="-%f", w779) -> (resulting string=w776:string)  [unwired: 2 in, 1 out]
                        n504 = global write "Global 1.vi" "X_havetogo"(w776) -> ()
                      }
                    }
                    n505 = global read "Global 1.vi" "RX_부호"() -> (w765:string)
                    n506 = global read "Global 1.vi" "RZ_부호"() -> (w763:string)
                    n507 = global read "Global 1.vi" "RY_부호"() -> (w764:string)
                    n508 = case shown="\"1\"" w763 {
                      frame "False", Default {
                      }
                      frame "True" {
                      }
                      frame "2" {
                      }
                      frame "1" {
                        n509 = global read "Global 1.vi" "RZ_havetogo"() -> (w782:string)
                        n510 = Decimal String To Number(string=w782) -> (number=w785:i32)  [unwired: 2 in, 1 out]
                        n511 = To Double Precision Float(number=w785) -> (double precision float=w784:dbl)
                        n512 = Format Into String(format string="-%f", w784) -> (resulting string=w781:string)  [unwired: 2 in, 1 out]
                        n513 = global write "Global 1.vi" "RZ_havetogo"(w781) -> ()
                      }
                    }
                    n514 = case shown="\"1\"" w764 {
                      frame "False", Default {
                      }
                      frame "True" {
                      }
                      frame "2" {
                      }
                      frame "1" {
                        n515 = global read "Global 1.vi" "RY_havetogo"() -> (w787:string)
                        n516 = Decimal String To Number(string=w787) -> (number=w790:i32)  [unwired: 2 in, 1 out]
                        n517 = To Double Precision Float(number=w790) -> (double precision float=w788:dbl)
                        n518 = Format Into String(format string="-%f", w788) -> (resulting string=w786:string)  [unwired: 2 in, 1 out]
                        n519 = global write "Global 1.vi" "RY_havetogo"(w786) -> ()
                      }
                    }
                    n520 = case shown="\"1\"" w765 {
                      frame "False", Default {
                      }
                      frame "True" {
                      }
                      frame "2" {
                      }
                      frame "1" {
                        n521 = global read "Global 1.vi" "RX_havetogo"() -> (w792:string)
                        n522 = Decimal String To Number(string=w792) -> (number=w795:i32)  [unwired: 2 in, 1 out]
                        n523 = To Double Precision Float(number=w795) -> (double precision float=w794:dbl)
                        n524 = Format Into String(format string="-%f", w794) -> (resulting string=w791:string)  [unwired: 2 in, 1 out]
                        n525 = global write "Global 1.vi" "RX_havetogo"(w791) -> ()
                      }
                    }
                  }
                  frame #1 {
                    n526 = global read "Global 1.vi" "X_havetogo"() -> (w807:string)
                    n527 = global read "Global 1.vi" "Y_havetogo"() -> (w806:string)
                    n528 = global read "Global 1.vi" "Z_havetogo"() -> (w805:string)
                    n529 = global read "Global 1.vi" "RX_havetogo"() -> (w804:string)
                    n530 = global read "Global 1.vi" "RY_havetogo"() -> (w803:string)
                    n531 = global read "Global 1.vi" "RZ_havetogo"() -> (w802:string)
                    n532 = Decimal String To Number(string=w805) -> (number=w831:i32)  [unwired: 2 in, 1 out]
                    n533 = Decimal String To Number(string=w807) -> (number=w837:i32)  [unwired: 2 in, 1 out]
                    n534 = Decimal String To Number(string=w806) -> (number=w834:i32)  [unwired: 2 in, 1 out]
                    n535 = Decimal String To Number(string=w804) -> (number=w828:i32)  [unwired: 2 in, 1 out]
                    n536 = Decimal String To Number(string=w803) -> (number=w825:i32)  [unwired: 2 in, 1 out]
                    n537 = Decimal String To Number(string=w802) -> (number=w822:i32)  [unwired: 2 in, 1 out]
                    n538 = To Double Precision Float(number=w831) -> (double precision float=w833:dbl)
                    n539 = To Double Precision Float(number=w837) -> (double precision float=w839:dbl)
                    n540 = To Double Precision Float(number=w834) -> (double precision float=w836:dbl)
                    n541 = To Double Precision Float(number=w828) -> (double precision float=w830:dbl)
                    n542 = To Double Precision Float(number=w825) -> (double precision float=w827:dbl)
                    n543 = Multiply(x=w839, y=0.001) -> (x*y=w821:dbl)
                    n544 = Multiply(x=w833, y=0.001) -> (x*y=w817:dbl)
                    n545 = Multiply(x=w836, y=0.001) -> (x*y=w819:dbl)
                    n546 = Multiply(x=w830, y=0.001) -> (x*y=w815:dbl)
                    n547 = global read "Global 1.vi" "x"() -> (w801:dbl)
                    n548 = Multiply(x=w827, y=0.001) -> (x*y=w813:dbl)
                    n549 = global read "Global 1.vi" "y"() -> (w800:dbl)
                    n550 = global read "Global 1.vi" "rx"() -> (w798:dbl)
                    n551 = global read "Global 1.vi" "z"() -> (w799:dbl)
                    n552 = To Double Precision Float(number=w822) -> (double precision float=w824:dbl)
                    n553 = Add(x=w801, y=w821) -> (x+y=w820:dbl)
                    n554 = Multiply(x=w824, y=0.001) -> (x*y=w811:dbl)
                    n555 = Add(x=w817, y=w799) -> (x+y=w816:dbl)
                    n556 = Add(x=w819, y=w800) -> (x+y=w818:dbl)
                    n557 = global read "Global 1.vi" "ry"() -> (w796:dbl)
                    n558 = global read "Global 1.vi" "rz"() -> (w797:dbl)
                    n559 = Add(x=w815, y=w798) -> (x+y=w814:dbl)
                    n560 = Add(x=w813, y=w796) -> (x+y=w812:dbl)
                    n561 = Add(x=w811, y=w797) -> (x+y=w810:dbl)
                    n562 = Format Into String(format string="movej( get_inverse_kin(p[%f, %f, %f, %f, %f, %f]), a= 0.5, v=0.25, t=0, r=0)", w820, w818, w816, w814, w812, w810) -> (resulting string=w808:string)  [unwired: 2 in, 1 out]
                    n563 = global write "Global 1.vi" "잭다니엘 카메라 값"(w808) -> ()
                  }
                }
              }
              frame "1" {
                n564 = flat-sequence {
                  frame #0 {
                    n565 = global read "Global 1.vi" "X_부호"() -> (w842:string)
                    n566 = global read "Global 1.vi" "Z_부호"() -> (w840:string)
                    n567 = global read "Global 1.vi" "Y_부호"() -> (w841:string)
                    n568 = case shown="\"1\"" w840 {
                      frame "False", Default {
                      }
                      frame "True" {
                      }
                      frame "2" {
                      }
                      frame "1" {
                        n569 = global read "Global 1.vi" "Z_havetogo"() -> (w847:string)
                        n570 = Decimal String To Number(string=w847) -> (number=w850:i32)  [unwired: 2 in, 1 out]
                        n571 = To Double Precision Float(number=w850) -> (double precision float=w849:dbl)
                        n572 = Format Into String(format string="-%f", w849) -> (resulting string=w846:string)  [unwired: 2 in, 1 out]
                        n573 = global write "Global 1.vi" "Z_havetogo"(w846) -> ()
                      }
                    }
                    n574 = case shown="\"1\"" w841 {
                      frame "False", Default {
                      }
                      frame "True" {
                      }
                      frame "2" {
                      }
                      frame "1" {
                        n575 = global read "Global 1.vi" "Y_havetogo"() -> (w852:string)
                        n576 = Decimal String To Number(string=w852) -> (number=w855:i32)  [unwired: 2 in, 1 out]
                        n577 = To Double Precision Float(number=w855) -> (double precision float=w853:dbl)
                        n578 = Format Into String(format string="-%f", w853) -> (resulting string=w851:string)  [unwired: 2 in, 1 out]
                        n579 = global write "Global 1.vi" "Y_havetogo"(w851) -> ()
                      }
                    }
                    n580 = case shown="\"1\"" w842 {
                      frame "False", Default {
                      }
                      frame "True" {
                      }
                      frame "2" {
                      }
                      frame "1" {
                        n581 = global read "Global 1.vi" "X_havetogo"() -> (w857:string)
                        n582 = Decimal String To Number(string=w857) -> (number=w860:i32)  [unwired: 2 in, 1 out]
                        n583 = To Double Precision Float(number=w860) -> (double precision float=w859:dbl)
                        n584 = Format Into String(format string="-%f", w859) -> (resulting string=w856:string)  [unwired: 2 in, 1 out]
                        n585 = global write "Global 1.vi" "X_havetogo"(w856) -> ()
                      }
                    }
                    n586 = global read "Global 1.vi" "RX_부호"() -> (w845:string)
                    n587 = global read "Global 1.vi" "RZ_부호"() -> (w843:string)
                    n588 = global read "Global 1.vi" "RY_부호"() -> (w844:string)
                    n589 = case shown="\"1\"" w843 {
                      frame "False", Default {
                      }
                      frame "True" {
                      }
                      frame "2" {
                      }
                      frame "1" {
                        n590 = global read "Global 1.vi" "RZ_havetogo"() -> (w862:string)
                        n591 = Decimal String To Number(string=w862) -> (number=w865:i32)  [unwired: 2 in, 1 out]
                        n592 = To Double Precision Float(number=w865) -> (double precision float=w864:dbl)
                        n593 = Format Into String(format string="-%f", w864) -> (resulting string=w861:string)  [unwired: 2 in, 1 out]
                        n594 = global write "Global 1.vi" "RZ_havetogo"(w861) -> ()
                      }
                    }
                    n595 = case shown="\"1\"" w844 {
                      frame "False", Default {
                      }
                      frame "True" {
                      }
                      frame "2" {
                      }
                      frame "1" {
                        n596 = global read "Global 1.vi" "RY_havetogo"() -> (w867:string)
                        n597 = Decimal String To Number(string=w867) -> (number=w870:i32)  [unwired: 2 in, 1 out]
                        n598 = To Double Precision Float(number=w870) -> (double precision float=w868:dbl)
                        n599 = Format Into String(format string="-%f", w868) -> (resulting string=w866:string)  [unwired: 2 in, 1 out]
                        n600 = global write "Global 1.vi" "RY_havetogo"(w866) -> ()
                      }
                    }
                    n601 = case shown="\"1\"" w845 {
                      frame "False", Default {
                      }
                      frame "True" {
                      }
                      frame "2" {
                      }
                      frame "1" {
                        n602 = global read "Global 1.vi" "RX_havetogo"() -> (w872:string)
                        n603 = Decimal String To Number(string=w872) -> (number=w875:i32)  [unwired: 2 in, 1 out]
                        n604 = To Double Precision Float(number=w875) -> (double precision float=w874:dbl)
                        n605 = Format Into String(format string="-%f", w874) -> (resulting string=w871:string)  [unwired: 2 in, 1 out]
                        n606 = global write "Global 1.vi" "RX_havetogo"(w871) -> ()
                      }
                    }
                  }
                  frame #1 {
                    n607 = global read "Global 1.vi" "X_havetogo"() -> (w887:string)
                    n608 = global read "Global 1.vi" "Y_havetogo"() -> (w886:string)
                    n609 = global read "Global 1.vi" "Z_havetogo"() -> (w885:string)
                    n610 = global read "Global 1.vi" "RX_havetogo"() -> (w884:string)
                    n611 = global read "Global 1.vi" "RY_havetogo"() -> (w883:string)
                    n612 = global read "Global 1.vi" "RZ_havetogo"() -> (w882:string)
                    n613 = Decimal String To Number(string=w885) -> (number=w911:i32)  [unwired: 2 in, 1 out]
                    n614 = Decimal String To Number(string=w887) -> (number=w917:i32)  [unwired: 2 in, 1 out]
                    n615 = Decimal String To Number(string=w886) -> (number=w914:i32)  [unwired: 2 in, 1 out]
                    n616 = Decimal String To Number(string=w884) -> (number=w908:i32)  [unwired: 2 in, 1 out]
                    n617 = Decimal String To Number(string=w883) -> (number=w905:i32)  [unwired: 2 in, 1 out]
                    n618 = Decimal String To Number(string=w882) -> (number=w902:i32)  [unwired: 2 in, 1 out]
                    n619 = To Double Precision Float(number=w911) -> (double precision float=w913:dbl)
                    n620 = To Double Precision Float(number=w917) -> (double precision float=w919:dbl)
                    n621 = To Double Precision Float(number=w914) -> (double precision float=w916:dbl)
                    n622 = To Double Precision Float(number=w908) -> (double precision float=w910:dbl)
                    n623 = To Double Precision Float(number=w905) -> (double precision float=w907:dbl)
                    n624 = Multiply(x=w919, y=0.001) -> (x*y=w901:dbl)
                    n625 = Multiply(x=w913, y=0.001) -> (x*y=w897:dbl)
                    n626 = Multiply(x=w916, y=0.001) -> (x*y=w899:dbl)
                    n627 = Multiply(x=w910, y=0.001) -> (x*y=w895:dbl)
                    n628 = global read "Global 1.vi" "x"() -> (w881:dbl)
                    n629 = Multiply(x=w907, y=0.001) -> (x*y=w893:dbl)
                    n630 = global read "Global 1.vi" "y"() -> (w880:dbl)
                    n631 = global read "Global 1.vi" "rx"() -> (w878:dbl)
                    n632 = global read "Global 1.vi" "z"() -> (w879:dbl)
                    n633 = To Double Precision Float(number=w902) -> (double precision float=w904:dbl)
                    n634 = Add(x=w881, y=w901) -> (x+y=w900:dbl)
                    n635 = Multiply(x=w904, y=0.001) -> (x*y=w891:dbl)
                    n636 = Add(x=w897, y=w879) -> (x+y=w896:dbl)
                    n637 = Add(x=w899, y=w880) -> (x+y=w898:dbl)
                    n638 = global read "Global 1.vi" "ry"() -> (w876:dbl)
                    n639 = global read "Global 1.vi" "rz"() -> (w877:dbl)
                    n640 = Add(x=w895, y=w878) -> (x+y=w894:dbl)
                    n641 = Add(x=w893, y=w876) -> (x+y=w892:dbl)
                    n642 = Add(x=w891, y=w877) -> (x+y=w890:dbl)
                    n643 = Format Into String(format string="movej( get_inverse_kin(p[%f, %f, %f, %f, %f, %f]), a= 0.5, v=0.25, t=0, r=0)", w900, w898, w896, w894, w892, w890) -> (resulting string=w888:string)  [unwired: 2 in, 1 out]
                    n644 = global write "Global 1.vi" "우유 카메라 값"(w888) -> ()
                  }
                }
              }
              frame "2" {
                n645 = flat-sequence {
                  frame #0 {
                    n646 = global read "Global 1.vi" "X_부호"() -> (w922:string)
                    n647 = global read "Global 1.vi" "Z_부호"() -> (w920:string)
                    n648 = global read "Global 1.vi" "Y_부호"() -> (w921:string)
                    n649 = case shown="\"1\"" w920 {
                      frame "False", Default {
                      }
                      frame "True" {
                      }
                      frame "2" {
                      }
                      frame "1" {
                        n650 = global read "Global 1.vi" "Z_havetogo"() -> (w927:string)
                        n651 = Decimal String To Number(string=w927) -> (number=w930:i32)  [unwired: 2 in, 1 out]
                        n652 = To Double Precision Float(number=w930) -> (double precision float=w929:dbl)
                        n653 = Format Into String(format string="-%f", w929) -> (resulting string=w926:string)  [unwired: 2 in, 1 out]
                        n654 = global write "Global 1.vi" "Z_havetogo"(w926) -> ()
                      }
                    }
                    n655 = case shown="\"1\"" w921 {
                      frame "False", Default {
                      }
                      frame "True" {
                      }
                      frame "2" {
                      }
                      frame "1" {
                        n656 = global read "Global 1.vi" "Y_havetogo"() -> (w932:string)
                        n657 = Decimal String To Number(string=w932) -> (number=w935:i32)  [unwired: 2 in, 1 out]
                        n658 = To Double Precision Float(number=w935) -> (double precision float=w933:dbl)
                        n659 = Format Into String(format string="-%f", w933) -> (resulting string=w931:string)  [unwired: 2 in, 1 out]
                        n660 = global write "Global 1.vi" "Y_havetogo"(w931) -> ()
                      }
                    }
                    n661 = case shown="\"1\"" w922 {
                      frame "False", Default {
                      }
                      frame "True" {
                      }
                      frame "2" {
                      }
                      frame "1" {
                        n662 = global read "Global 1.vi" "X_havetogo"() -> (w937:string)
                        n663 = Decimal String To Number(string=w937) -> (number=w940:i32)  [unwired: 2 in, 1 out]
                        n664 = To Double Precision Float(number=w940) -> (double precision float=w939:dbl)
                        n665 = Format Into String(format string="-%f", w939) -> (resulting string=w936:string)  [unwired: 2 in, 1 out]
                        n666 = global write "Global 1.vi" "X_havetogo"(w936) -> ()
                      }
                    }
                    n667 = global read "Global 1.vi" "RX_부호"() -> (w925:string)
                    n668 = global read "Global 1.vi" "RZ_부호"() -> (w923:string)
                    n669 = global read "Global 1.vi" "RY_부호"() -> (w924:string)
                    n670 = case shown="\"1\"" w923 {
                      frame "False", Default {
                      }
                      frame "True" {
                      }
                      frame "2" {
                      }
                      frame "1" {
                        n671 = global read "Global 1.vi" "RZ_havetogo"() -> (w942:string)
                        n672 = Decimal String To Number(string=w942) -> (number=w945:i32)  [unwired: 2 in, 1 out]
                        n673 = To Double Precision Float(number=w945) -> (double precision float=w944:dbl)
                        n674 = Format Into String(format string="-%f", w944) -> (resulting string=w941:string)  [unwired: 2 in, 1 out]
                        n675 = global write "Global 1.vi" "RZ_havetogo"(w941) -> ()
                      }
                    }
                    n676 = case shown="\"1\"" w924 {
                      frame "False", Default {
                      }
                      frame "True" {
                      }
                      frame "2" {
                      }
                      frame "1" {
                        n677 = global read "Global 1.vi" "RY_havetogo"() -> (w947:string)
                        n678 = Decimal String To Number(string=w947) -> (number=w950:i32)  [unwired: 2 in, 1 out]
                        n679 = To Double Precision Float(number=w950) -> (double precision float=w948:dbl)
                        n680 = Format Into String(format string="-%f", w948) -> (resulting string=w946:string)  [unwired: 2 in, 1 out]
                        n681 = global write "Global 1.vi" "RY_havetogo"(w946) -> ()
                      }
                    }
                    n682 = case shown="\"1\"" w925 {
                      frame "False", Default {
                      }
                      frame "True" {
                      }
                      frame "2" {
                      }
                      frame "1" {
                        n683 = global read "Global 1.vi" "RX_havetogo"() -> (w952:string)
                        n684 = Decimal String To Number(string=w952) -> (number=w955:i32)  [unwired: 2 in, 1 out]
                        n685 = To Double Precision Float(number=w955) -> (double precision float=w954:dbl)
                        n686 = Format Into String(format string="-%f", w954) -> (resulting string=w951:string)  [unwired: 2 in, 1 out]
                        n687 = global write "Global 1.vi" "RX_havetogo"(w951) -> ()
                      }
                    }
                  }
                  frame #1 {
                    n688 = global read "Global 1.vi" "X_havetogo"() -> (w967:string)
                    n689 = global read "Global 1.vi" "Y_havetogo"() -> (w966:string)
                    n690 = global read "Global 1.vi" "Z_havetogo"() -> (w965:string)
                    n691 = global read "Global 1.vi" "RX_havetogo"() -> (w964:string)
                    n692 = global read "Global 1.vi" "RY_havetogo"() -> (w963:string)
                    n693 = global read "Global 1.vi" "RZ_havetogo"() -> (w962:string)
                    n694 = Decimal String To Number(string=w965) -> (number=w991:i32)  [unwired: 2 in, 1 out]
                    n695 = Decimal String To Number(string=w967) -> (number=w997:i32)  [unwired: 2 in, 1 out]
                    n696 = Decimal String To Number(string=w966) -> (number=w994:i32)  [unwired: 2 in, 1 out]
                    n697 = Decimal String To Number(string=w964) -> (number=w988:i32)  [unwired: 2 in, 1 out]
                    n698 = Decimal String To Number(string=w963) -> (number=w985:i32)  [unwired: 2 in, 1 out]
                    n699 = Decimal String To Number(string=w962) -> (number=w982:i32)  [unwired: 2 in, 1 out]
                    n700 = To Double Precision Float(number=w991) -> (double precision float=w993:dbl)
                    n701 = To Double Precision Float(number=w997) -> (double precision float=w999:dbl)
                    n702 = To Double Precision Float(number=w994) -> (double precision float=w996:dbl)
                    n703 = To Double Precision Float(number=w988) -> (double precision float=w990:dbl)
                    n704 = To Double Precision Float(number=w985) -> (double precision float=w987:dbl)
                    n705 = Multiply(x=w999, y=0.001) -> (x*y=w981:dbl)
                    n706 = Multiply(x=w993, y=0.001) -> (x*y=w977:dbl)
                    n707 = Multiply(x=w996, y=0.001) -> (x*y=w979:dbl)
                    n708 = Multiply(x=w990, y=0.001) -> (x*y=w975:dbl)
                    n709 = global read "Global 1.vi" "x"() -> (w961:dbl)
                    n710 = Multiply(x=w987, y=0.001) -> (x*y=w973:dbl)
                    n711 = global read "Global 1.vi" "y"() -> (w960:dbl)
                    n712 = global read "Global 1.vi" "rx"() -> (w958:dbl)
                    n713 = global read "Global 1.vi" "z"() -> (w959:dbl)
                    n714 = To Double Precision Float(number=w982) -> (double precision float=w984:dbl)
                    n715 = Add(x=w961, y=w981) -> (x+y=w980:dbl)
                    n716 = Multiply(x=w984, y=0.001) -> (x*y=w971:dbl)
                    n717 = Add(x=w977, y=w959) -> (x+y=w976:dbl)
                    n718 = Add(x=w979, y=w960) -> (x+y=w978:dbl)
                    n719 = global read "Global 1.vi" "ry"() -> (w956:dbl)
                    n720 = global read "Global 1.vi" "rz"() -> (w957:dbl)
                    n721 = Add(x=w975, y=w958) -> (x+y=w974:dbl)
                    n722 = Add(x=w973, y=w956) -> (x+y=w972:dbl)
                    n723 = Add(x=w971, y=w957) -> (x+y=w970:dbl)
                    n724 = Format Into String(format string="movej( get_inverse_kin(p[%f, %f, %f, %f, %f, %f]), a= 0.5, v=0.25, t=0, r=0)", w980, w978, w976, w974, w972, w970) -> (resulting string=w968:string)  [unwired: 2 in, 1 out]
                    n725 = global write "Global 1.vi" "짐빔 카메라 값"(w968) -> ()
                  }
                }
              }
              frame "3" {
                n726 = flat-sequence {
                  frame #0 {
                    n727 = global read "Global 1.vi" "X_부호"() -> (w1002:string)
                    n728 = global read "Global 1.vi" "Z_부호"() -> (w1000:string)
                    n729 = global read "Global 1.vi" "Y_부호"() -> (w1001:string)
                    n730 = case shown="\"1\"" w1000 {
                      frame "False", Default {
                      }
                      frame "True" {
                      }
                      frame "2" {
                      }
                      frame "1" {
                        n731 = global read "Global 1.vi" "Z_havetogo"() -> (w1007:string)
                        n732 = Decimal String To Number(string=w1007) -> (number=w1010:i32)  [unwired: 2 in, 1 out]
                        n733 = To Double Precision Float(number=w1010) -> (double precision float=w1009:dbl)
                        n734 = Format Into String(format string="-%f", w1009) -> (resulting string=w1006:string)  [unwired: 2 in, 1 out]
                        n735 = global write "Global 1.vi" "Z_havetogo"(w1006) -> ()
                      }
                    }
                    n736 = case shown="\"1\"" w1001 {
                      frame "False", Default {
                      }
                      frame "True" {
                      }
                      frame "2" {
                      }
                      frame "1" {
                        n737 = global read "Global 1.vi" "Y_havetogo"() -> (w1012:string)
                        n738 = Decimal String To Number(string=w1012) -> (number=w1015:i32)  [unwired: 2 in, 1 out]
                        n739 = To Double Precision Float(number=w1015) -> (double precision float=w1013:dbl)
                        n740 = Format Into String(format string="-%f", w1013) -> (resulting string=w1011:string)  [unwired: 2 in, 1 out]
                        n741 = global write "Global 1.vi" "Y_havetogo"(w1011) -> ()
                      }
                    }
                    n742 = case shown="\"1\"" w1002 {
                      frame "False", Default {
                      }
                      frame "True" {
                      }
                      frame "2" {
                      }
                      frame "1" {
                        n743 = global read "Global 1.vi" "X_havetogo"() -> (w1017:string)
                        n744 = Decimal String To Number(string=w1017) -> (number=w1020:i32)  [unwired: 2 in, 1 out]
                        n745 = To Double Precision Float(number=w1020) -> (double precision float=w1019:dbl)
                        n746 = Format Into String(format string="-%f", w1019) -> (resulting string=w1016:string)  [unwired: 2 in, 1 out]
                        n747 = global write "Global 1.vi" "X_havetogo"(w1016) -> ()
                      }
                    }
                    n748 = global read "Global 1.vi" "RX_부호"() -> (w1005:string)
                    n749 = global read "Global 1.vi" "RZ_부호"() -> (w1003:string)
                    n750 = global read "Global 1.vi" "RY_부호"() -> (w1004:string)
                    n751 = case shown="\"1\"" w1003 {
                      frame "False", Default {
                      }
                      frame "True" {
                      }
                      frame "2" {
                      }
                      frame "1" {
                        n752 = global read "Global 1.vi" "RZ_havetogo"() -> (w1022:string)
                        n753 = Decimal String To Number(string=w1022) -> (number=w1025:i32)  [unwired: 2 in, 1 out]
                        n754 = To Double Precision Float(number=w1025) -> (double precision float=w1024:dbl)
                        n755 = Format Into String(format string="-%f", w1024) -> (resulting string=w1021:string)  [unwired: 2 in, 1 out]
                        n756 = global write "Global 1.vi" "RZ_havetogo"(w1021) -> ()
                      }
                    }
                    n757 = case shown="\"1\"" w1004 {
                      frame "False", Default {
                      }
                      frame "True" {
                      }
                      frame "2" {
                      }
                      frame "1" {
                        n758 = global read "Global 1.vi" "RY_havetogo"() -> (w1027:string)
                        n759 = Decimal String To Number(string=w1027) -> (number=w1030:i32)  [unwired: 2 in, 1 out]
                        n760 = To Double Precision Float(number=w1030) -> (double precision float=w1028:dbl)
                        n761 = Format Into String(format string="-%f", w1028) -> (resulting string=w1026:string)  [unwired: 2 in, 1 out]
                        n762 = global write "Global 1.vi" "RY_havetogo"(w1026) -> ()
                      }
                    }
                    n763 = case shown="\"1\"" w1005 {
                      frame "False", Default {
                      }
                      frame "True" {
                      }
                      frame "2" {
                      }
                      frame "1" {
                        n764 = global read "Global 1.vi" "RX_havetogo"() -> (w1032:string)
                        n765 = Decimal String To Number(string=w1032) -> (number=w1035:i32)  [unwired: 2 in, 1 out]
                        n766 = To Double Precision Float(number=w1035) -> (double precision float=w1034:dbl)
                        n767 = Format Into String(format string="-%f", w1034) -> (resulting string=w1031:string)  [unwired: 2 in, 1 out]
                        n768 = global write "Global 1.vi" "RX_havetogo"(w1031) -> ()
                      }
                    }
                  }
                  frame #1 {
                    n769 = global read "Global 1.vi" "X_havetogo"() -> (w1047:string)
                    n770 = global read "Global 1.vi" "Y_havetogo"() -> (w1046:string)
                    n771 = global read "Global 1.vi" "Z_havetogo"() -> (w1045:string)
                    n772 = global read "Global 1.vi" "RX_havetogo"() -> (w1044:string)
                    n773 = global read "Global 1.vi" "RY_havetogo"() -> (w1043:string)
                    n774 = global read "Global 1.vi" "RZ_havetogo"() -> (w1042:string)
                    n775 = Decimal String To Number(string=w1045) -> (number=w1071:i32)  [unwired: 2 in, 1 out]
                    n776 = Decimal String To Number(string=w1047) -> (number=w1077:i32)  [unwired: 2 in, 1 out]
                    n777 = Decimal String To Number(string=w1046) -> (number=w1074:i32)  [unwired: 2 in, 1 out]
                    n778 = Decimal String To Number(string=w1044) -> (number=w1068:i32)  [unwired: 2 in, 1 out]
                    n779 = Decimal String To Number(string=w1043) -> (number=w1065:i32)  [unwired: 2 in, 1 out]
                    n780 = Decimal String To Number(string=w1042) -> (number=w1062:i32)  [unwired: 2 in, 1 out]
                    n781 = To Double Precision Float(number=w1071) -> (double precision float=w1073:dbl)
                    n782 = To Double Precision Float(number=w1077) -> (double precision float=w1079:dbl)
                    n783 = To Double Precision Float(number=w1074) -> (double precision float=w1076:dbl)
                    n784 = To Double Precision Float(number=w1068) -> (double precision float=w1070:dbl)
                    n785 = To Double Precision Float(number=w1065) -> (double precision float=w1067:dbl)
                    n786 = Multiply(x=w1079, y=0.001) -> (x*y=w1061:dbl)
                    n787 = Multiply(x=w1073, y=0.001) -> (x*y=w1057:dbl)
                    n788 = Multiply(x=w1076, y=0.001) -> (x*y=w1059:dbl)
                    n789 = Multiply(x=w1070, y=0.001) -> (x*y=w1055:dbl)
                    n790 = global read "Global 1.vi" "x"() -> (w1041:dbl)
                    n791 = Multiply(x=w1067, y=0.001) -> (x*y=w1053:dbl)
                    n792 = global read "Global 1.vi" "y"() -> (w1040:dbl)
                    n793 = global read "Global 1.vi" "rx"() -> (w1038:dbl)
                    n794 = global read "Global 1.vi" "z"() -> (w1039:dbl)
                    n795 = To Double Precision Float(number=w1062) -> (double precision float=w1064:dbl)
                    n796 = Add(x=w1041, y=w1061) -> (x+y=w1060:dbl)
                    n797 = Multiply(x=w1064, y=0.001) -> (x*y=w1051:dbl)
                    n798 = Add(x=w1057, y=w1039) -> (x+y=w1056:dbl)
                    n799 = Add(x=w1059, y=w1040) -> (x+y=w1058:dbl)
                    n800 = global read "Global 1.vi" "ry"() -> (w1036:dbl)
                    n801 = global read "Global 1.vi" "rz"() -> (w1037:dbl)
                    n802 = Add(x=w1055, y=w1038) -> (x+y=w1054:dbl)
                    n803 = Add(x=w1053, y=w1036) -> (x+y=w1052:dbl)
                    n804 = Add(x=w1051, y=w1037) -> (x+y=w1050:dbl)
                    n805 = Format Into String(format string="movej( get_inverse_kin(p[%f, %f, %f, %f, %f, %f]), a= 0.5, v=0.25, t=0, r=0)", w1060, w1058, w1056, w1054, w1052, w1050) -> (resulting string=w1048:string)  [unwired: 2 in, 1 out]
                    n806 = global write "Global 1.vi" "토닉 카메라 값"(w1048) -> ()
                  }
                }
              }
              frame "4" {
                n807 = flat-sequence {
                  frame #0 {
                    n808 = global read "Global 1.vi" "X_부호"() -> (w1082:string)
                    n809 = global read "Global 1.vi" "Z_부호"() -> (w1080:string)
                    n810 = global read "Global 1.vi" "Y_부호"() -> (w1081:string)
                    n811 = case shown="\"1\"" w1080 {
                      frame "False", Default {
                      }
                      frame "True" {
                      }
                      frame "2" {
                      }
                      frame "1" {
                        n812 = global read "Global 1.vi" "Z_havetogo"() -> (w1087:string)
                        n813 = Decimal String To Number(string=w1087) -> (number=w1090:i32)  [unwired: 2 in, 1 out]
                        n814 = To Double Precision Float(number=w1090) -> (double precision float=w1089:dbl)
                        n815 = Format Into String(format string="-%f", w1089) -> (resulting string=w1086:string)  [unwired: 2 in, 1 out]
                        n816 = global write "Global 1.vi" "Z_havetogo"(w1086) -> ()
                      }
                    }
                    n817 = case shown="\"1\"" w1081 {
                      frame "False", Default {
                      }
                      frame "True" {
                      }
                      frame "2" {
                      }
                      frame "1" {
                        n818 = global read "Global 1.vi" "Y_havetogo"() -> (w1092:string)
                        n819 = Decimal String To Number(string=w1092) -> (number=w1095:i32)  [unwired: 2 in, 1 out]
                        n820 = To Double Precision Float(number=w1095) -> (double precision float=w1093:dbl)
                        n821 = Format Into String(format string="-%f", w1093) -> (resulting string=w1091:string)  [unwired: 2 in, 1 out]
                        n822 = global write "Global 1.vi" "Y_havetogo"(w1091) -> ()
                      }
                    }
                    n823 = case shown="\"1\"" w1082 {
                      frame "False", Default {
                      }
                      frame "True" {
                      }
                      frame "2" {
                      }
                      frame "1" {
                        n824 = global read "Global 1.vi" "X_havetogo"() -> (w1097:string)
                        n825 = Decimal String To Number(string=w1097) -> (number=w1100:i32)  [unwired: 2 in, 1 out]
                        n826 = To Double Precision Float(number=w1100) -> (double precision float=w1099:dbl)
                        n827 = Format Into String(format string="-%f", w1099) -> (resulting string=w1096:string)  [unwired: 2 in, 1 out]
                        n828 = global write "Global 1.vi" "X_havetogo"(w1096) -> ()
                      }
                    }
                    n829 = global read "Global 1.vi" "RX_부호"() -> (w1085:string)
                    n830 = global read "Global 1.vi" "RZ_부호"() -> (w1083:string)
                    n831 = global read "Global 1.vi" "RY_부호"() -> (w1084:string)
                    n832 = case shown="\"1\"" w1083 {
                      frame "False", Default {
                      }
                      frame "True" {
                      }
                      frame "2" {
                      }
                      frame "1" {
                        n833 = global read "Global 1.vi" "RZ_havetogo"() -> (w1102:string)
                        n834 = Decimal String To Number(string=w1102) -> (number=w1105:i32)  [unwired: 2 in, 1 out]
                        n835 = To Double Precision Float(number=w1105) -> (double precision float=w1104:dbl)
                        n836 = Format Into String(format string="-%f", w1104) -> (resulting string=w1101:string)  [unwired: 2 in, 1 out]
                        n837 = global write "Global 1.vi" "RZ_havetogo"(w1101) -> ()
                      }
                    }
                    n838 = case shown="\"1\"" w1084 {
                      frame "False", Default {
                      }
                      frame "True" {
                      }
                      frame "2" {
                      }
                      frame "1" {
                        n839 = global read "Global 1.vi" "RY_havetogo"() -> (w1107:string)
                        n840 = Decimal String To Number(string=w1107) -> (number=w1110:i32)  [unwired: 2 in, 1 out]
                        n841 = To Double Precision Float(number=w1110) -> (double precision float=w1108:dbl)
                        n842 = Format Into String(format string="-%f", w1108) -> (resulting string=w1106:string)  [unwired: 2 in, 1 out]
                        n843 = global write "Global 1.vi" "RY_havetogo"(w1106) -> ()
                      }
                    }
                    n844 = case shown="\"1\"" w1085 {
                      frame "False", Default {
                      }
                      frame "True" {
                      }
                      frame "2" {
                      }
                      frame "1" {
                        n845 = global read "Global 1.vi" "RX_havetogo"() -> (w1112:string)
                        n846 = Decimal String To Number(string=w1112) -> (number=w1115:i32)  [unwired: 2 in, 1 out]
                        n847 = To Double Precision Float(number=w1115) -> (double precision float=w1114:dbl)
                        n848 = Format Into String(format string="-%f", w1114) -> (resulting string=w1111:string)  [unwired: 2 in, 1 out]
                        n849 = global write "Global 1.vi" "RX_havetogo"(w1111) -> ()
                      }
                    }
                  }
                  frame #1 {
                    n850 = global read "Global 1.vi" "X_havetogo"() -> (w1127:string)
                    n851 = global read "Global 1.vi" "Y_havetogo"() -> (w1126:string)
                    n852 = global read "Global 1.vi" "Z_havetogo"() -> (w1125:string)
                    n853 = global read "Global 1.vi" "RX_havetogo"() -> (w1124:string)
                    n854 = global read "Global 1.vi" "RY_havetogo"() -> (w1123:string)
                    n855 = global read "Global 1.vi" "RZ_havetogo"() -> (w1122:string)
                    n856 = Decimal String To Number(string=w1125) -> (number=w1151:i32)  [unwired: 2 in, 1 out]
                    n857 = Decimal String To Number(string=w1127) -> (number=w1157:i32)  [unwired: 2 in, 1 out]
                    n858 = Decimal String To Number(string=w1126) -> (number=w1154:i32)  [unwired: 2 in, 1 out]
                    n859 = Decimal String To Number(string=w1124) -> (number=w1148:i32)  [unwired: 2 in, 1 out]
                    n860 = Decimal String To Number(string=w1123) -> (number=w1145:i32)  [unwired: 2 in, 1 out]
                    n861 = Decimal String To Number(string=w1122) -> (number=w1142:i32)  [unwired: 2 in, 1 out]
                    n862 = To Double Precision Float(number=w1151) -> (double precision float=w1153:dbl)
                    n863 = To Double Precision Float(number=w1157) -> (double precision float=w1159:dbl)
                    n864 = To Double Precision Float(number=w1154) -> (double precision float=w1156:dbl)
                    n865 = To Double Precision Float(number=w1148) -> (double precision float=w1150:dbl)
                    n866 = To Double Precision Float(number=w1145) -> (double precision float=w1147:dbl)
                    n867 = Multiply(x=w1159, y=0.001) -> (x*y=w1141:dbl)
                    n868 = Multiply(x=w1153, y=0.001) -> (x*y=w1137:dbl)
                    n869 = Multiply(x=w1156, y=0.001) -> (x*y=w1139:dbl)
                    n870 = Multiply(x=w1150, y=0.001) -> (x*y=w1135:dbl)
                    n871 = global read "Global 1.vi" "x"() -> (w1121:dbl)
                    n872 = Multiply(x=w1147, y=0.001) -> (x*y=w1133:dbl)
                    n873 = global read "Global 1.vi" "y"() -> (w1120:dbl)
                    n874 = global read "Global 1.vi" "rx"() -> (w1118:dbl)
                    n875 = global read "Global 1.vi" "z"() -> (w1119:dbl)
                    n876 = To Double Precision Float(number=w1142) -> (double precision float=w1144:dbl)
                    n877 = Add(x=w1121, y=w1141) -> (x+y=w1140:dbl)
                    n878 = Multiply(x=w1144, y=0.001) -> (x*y=w1131:dbl)
                    n879 = Add(x=w1137, y=w1119) -> (x+y=w1136:dbl)
                    n880 = Add(x=w1139, y=w1120) -> (x+y=w1138:dbl)
                    n881 = global read "Global 1.vi" "ry"() -> (w1116:dbl)
                    n882 = global read "Global 1.vi" "rz"() -> (w1117:dbl)
                    n883 = Add(x=w1135, y=w1118) -> (x+y=w1134:dbl)
                    n884 = Add(x=w1133, y=w1116) -> (x+y=w1132:dbl)
                    n885 = Add(x=w1131, y=w1117) -> (x+y=w1130:dbl)
                    n886 = Format Into String(format string="movej( get_inverse_kin(p[%f, %f, %f, %f, %f, %f]), a= 0.5, v=0.25, t=0, r=0)", w1140, w1138, w1136, w1134, w1132, w1130) -> (resulting string=w1128:string)  [unwired: 2 in, 1 out]
                    n887 = global write "Global 1.vi" "콜라 카메라 값"(w1128) -> ()
                  }
                }
              }
              frame "5" {
              }
            }
          }
          frame #2 {
            n888 = global write "Global 1.vi" "TCP 스위치"(FALSE ("그리퍼 열림")) -> ()
          }
        }
      }
    }
    n889 = Wait Until Next ms Multiple(millisecond multiple=u32 100) -> ()  [unwired: 1 out]
  }
